vi "03 Channel Tester.vi"(8 "error in (no error)":errorcluster, 11 "Mode":T1(ring)) -> (0 "error out":errorcluster, 2 "CDAQ Data Out":dbl[](array[numeric]))   [LabVIEW 2009]
uses:
  Hybrid Water Heater/Experiments/Sensor.ctl
  <vilib>/DAQmx/read.llb/DAQmx Read (Analog 2D DBL NChan NSamp).vi
  Global Test Variables DPT.vi
  <vilib>/Analysis/NI_AALBase.lvlib
panel:
  in  "CDAQ Data":dbl[](array[numeric])
  in  "Rate":dbl=1000.0
  out "Voltages":dbl[][](graph)
  in  "End":bool
  out "Analog Samples":i32
  in  "I.Bar":i32=5
  out "Bar":cluster{"Mean":dbl, "StdDev":dbl}
  in  "I.Gvol":i32=3
  out "G.Vol":cluster{"Mean":dbl, "StdDev":dbl}
  out "Weight":cluster{"Mean":dbl, "StdDev":dbl}
  in  "I.W":i32=1
  in  "I.Tmp":i32=4
  out "Temp":cluster{"Mean":dbl, "StdDev":dbl}
  out "RH":cluster{"Mean":dbl, "StdDev":dbl}
  in  "I.RH":i32=2
  out "G.Pres.":cluster{"Mean":dbl, "StdDev":dbl}
  in  "I.Gas Pressure":i32
  in  "Timeout":i32=1000
  out "Count":dbl
  out "error gather":errorcluster
  in  "Panel 4":T2[][](array[typedef])=[[{"Mean"=0.0, " Std"=0.0, "Color Box"=8585007}, {"Mean"=0.0, " Std"=0.0, "Color Box"=8585007}, {"Mean"=0.0, " Std"=0.0, "Color Box"=8585007}, {"Mean"=0.0, " Std"=0.0, "Color Box"=8585007}, {"Mean"=0.0, " Std"=0.0, "Color Box"=8585007}, {"Mean"=0.0, " Std"=0.0, "Color Box"=8585007}], [{"Mean"=0.0, " Std"=0.0, "Color Box"=8585007}, {"Mean"=0.0, " Std"=0.0, "Color Box"=8585007}, {"Mean"=0.0, " Std"=0.0, "Color Box"=8585007}, {"Mean"=0.0, " Std"=0.0, "Color Box"=8585007}, {"Mean"=0.0, " Std"=0.0, "Color Box"=8585007}, {"Mean"=0.0, " Std"=0.0, "Color Box"=8585007}], [{"Mean"=0.0, " Std"=0.0, "Color Box"=8585007}, {"Mean"=0.0, " Std"=0.0, "Color Box"=8585007}, {"Mean"=0.0, " Std"=0.0, "Color Box"=8585007}, {"Mean"=0.0, " Std"=0.0, "Color Box"=8585007}, {"Mean"=0.0, " Std"=0.0, "Color Box"=8585007}, {"Mean"=0.0, " Std"=0.0, "Color Box"=8585007}]]
  in  "StDev Thresh":dbl=0.2
  in  "TC Min OK Val":dbl=20.0
  in  "TC Max OK Val":dbl=400.0
  out "Gas Temp":T2={"Mean"=0.0, " Std"=0.0, "Color Box"=8585007}
  in  "Panel 3":T2[][](array[typedef])=[[{"Mean"=0.0, " Std"=0.0, "Color Box"=8585007}, {"Mean"=0.0, " Std"=0.0, "Color Box"=8585007}, {"Mean"=0.0, " Std"=0.0, "Color Box"=8585007}, {"Mean"=0.0, " Std"=0.0, "Color Box"=8585007}, {"Mean"=0.0, " Std"=0.0, "Color Box"=8585007}, {"Mean"=0.0, " Std"=0.0, "Color Box"=8585007}], [{"Mean"=0.0, " Std"=0.0, "Color Box"=8585007}, {"Mean"=0.0, " Std"=0.0, "Color Box"=8585007}, {"Mean"=0.0, " Std"=0.0, "Color Box"=8585007}, {"Mean"=0.0, " Std"=0.0, "Color Box"=8585007}, {"Mean"=0.0, " Std"=0.0, "Color Box"=8585007}, {"Mean"=0.0, " Std"=0.0, "Color Box"=8585007}], [{"Mean"=0.0, " Std"=0.0, "Color Box"=8585007}, {"Mean"=0.0, " Std"=0.0, "Color Box"=8585007}, {"Mean"=0.0, " Std"=0.0, "Color Box"=8585007}, {"Mean"=0.0, " Std"=0.0, "Color Box"=8585007}, {"Mean"=0.0, " Std"=0.0, "Color Box"=8585007}, {"Mean"=0.0, " Std"=0.0, "Color Box"=8585007}]]
  in  "Panel 2":T2[][](array[typedef])=[[{"Mean"=0.0, " Std"=0.0, "Color Box"=8585007}, {"Mean"=0.0, " Std"=0.0, "Color Box"=8585007}, {"Mean"=0.0, " Std"=0.0, "Color Box"=8585007}, {"Mean"=0.0, " Std"=0.0, "Color Box"=8585007}, {"Mean"=0.0, " Std"=0.0, "Color Box"=8585007}, {"Mean"=0.0, " Std"=0.0, "Color Box"=8585007}], [{"Mean"=0.0, " Std"=0.0, "Color Box"=8585007}, {"Mean"=0.0, " Std"=0.0, "Color Box"=8585007}, {"Mean"=0.0, " Std"=0.0, "Color Box"=8585007}, {"Mean"=0.0, " Std"=0.0, "Color Box"=8585007}, {"Mean"=0.0, " Std"=0.0, "Color Box"=8585007}, {"Mean"=0.0, " Std"=0.0, "Color Box"=8585007}], [{"Mean"=0.0, " Std"=0.0, "Color Box"=8585007}, {"Mean"=0.0, " Std"=0.0, "Color Box"=8585007}, {"Mean"=0.0, " Std"=0.0, "Color Box"=8585007}, {"Mean"=0.0, " Std"=0.0, "Color Box"=8585007}, {"Mean"=0.0, " Std"=0.0, "Color Box"=8585007}, {"Mean"=0.0, " Std"=0.0, "Color Box"=8585007}]]
  in  "Panel 1":T2[][](array[typedef])=[[{"Mean"=0.0, " Std"=0.0, "Color Box"=8585007}, {"Mean"=0.0, " Std"=0.0, "Color Box"=8585007}, {"Mean"=0.0, " Std"=0.0, "Color Box"=8585007}, {"Mean"=0.0, " Std"=0.0, "Color Box"=8585007}, {"Mean"=0.0, " Std"=0.0, "Color Box"=8585007}, {"Mean"=0.0, " Std"=0.0, "Color Box"=8585007}], [{"Mean"=0.0, " Std"=0.0, "Color Box"=8585007}, {"Mean"=0.0, " Std"=0.0, "Color Box"=8585007}, {"Mean"=0.0, " Std"=0.0, "Color Box"=8585007}, {"Mean"=0.0, " Std"=0.0, "Color Box"=8585007}, {"Mean"=0.0, " Std"=0.0, "Color Box"=8585007}, {"Mean"=0.0, " Std"=0.0, "Color Box"=8585007}], [{"Mean"=0.0, " Std"=0.0, "Color Box"=8585007}, {"Mean"=0.0, " Std"=0.0, "Color Box"=8585007}, {"Mean"=0.0, " Std"=0.0, "Color Box"=8585007}, {"Mean"=0.0, " Std"=0.0, "Color Box"=8585007}, {"Mean"=0.0, " Std"=0.0, "Color Box"=8585007}, {"Mean"=0.0, " Std"=0.0, "Color Box"=8585007}]]
  in  "Num Samples":i32=5
  in  "Test DAQ":bool
  in  "EXIT":bool
  # "DPT Pannel Channel Tester"
  # "Channel \nGas Pressure 0\nWeight 1\nRH 2\nGas Volume 3\nTemp 4\nBaromentric Pressure 5"
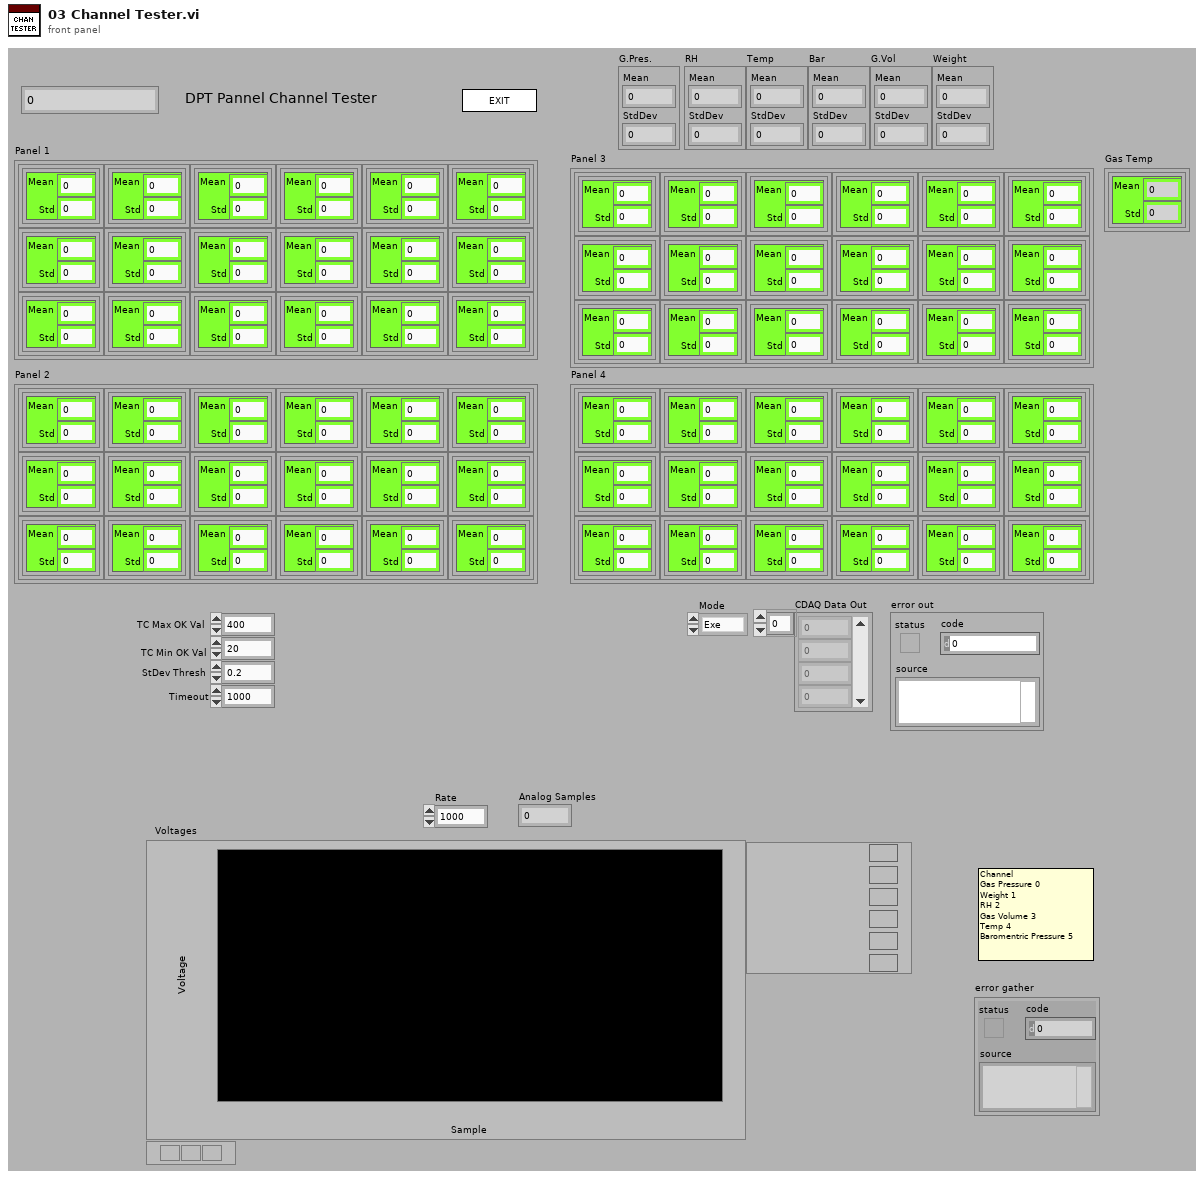
[diagram p1: front panel]
types:
  T1 = enum16{"Exe", "Init CDAQ", "Gather DATA", "Close"}
  T2 = typedef "Sensor.ctl" = cluster{"Mean":dbl, " Std":dbl, "Color Box":u32}
  T3 = enum32{"invalid app kind", "Development System", "Run Time System", "Student Edition", "Embedded LabVIEW", "Evaluation", "Custom"}
  T4 = enum32{"Invalid", "Standard", "Closed", "Hidden", "Minimized", "Maximized"}
  T5 = cluster{"Core":cluster{"Current VI Reference":refnum<vi>, "Close Panel on Exit?":bool}, "Num Samples":i32, "Temp task out":refnum<k21>, "Temp  Data Array":T2[], "AI task out":refnum<k21>, "AI Data":cluster{"Mean":dbl, "StdDev":dbl}[], "Init":bool, "CDAQ Data":dbl[]}
  T6 = cluster{"Current VI Reference":refnum<vi>, "Close Panel on Exit?":bool}
  T7 = typedef "DPT Global Type.ctl" = cluster{"Test Setup":cluster{"3010 resistor":dbl, "Temp Cal":dbl, "Temp Coeff":dbl, "Power On Threshold":dbl, "MA Filter Size":i32, "Weight Offset":dbl, "3011 resistor":dbl, "Gas Enabled":bool, "1020 resistor":dbl, "Scale Com":dbl, "W. Samps":i32}, "Agilent Setup":cluster{"Scale Channel":string, "TC Channels":string, "VDC Discrete Channels":string, "RH Chan":string, "Temp Chan":string, "Tscale Channel":string, "RDB Channel":string, "Gas Temperature":string, "Gas Pressure":string, "Barometric Pressure":string, "Gas Feedback Chan":string}, "Directories":cluster{"Work File Directory":path, "Save File Directory":path, "Library Directory":path, "Data Backup Directory":path}, "Test Information":cluster{"Model:":string, "Temperature:":string, "Engineer:":string, "Technician:":string, "Comments:":string, "Unit:":string, "TR Number:":string, "Test Number:":string, "Test Station:":string, "Empty Dryer Cold Weight:":dbl, "Serial Number:":string, "Build:":string, "Dryer Type":string, "Humidity":string, "Test Title per TR:":string}, "cDAQ Array Locations":cluster{"Scale Channel":string, "TC Channels":string, "VDC Discrete Channel":string, "RH Chan":string, "Temp Chan":string, "Tscale Channel":string, "RDB Channel":string, "Gas Temperature":string, "Gas Pressure":string, "Barometric Pressure":string, "Gas Feedback Chan":string}}
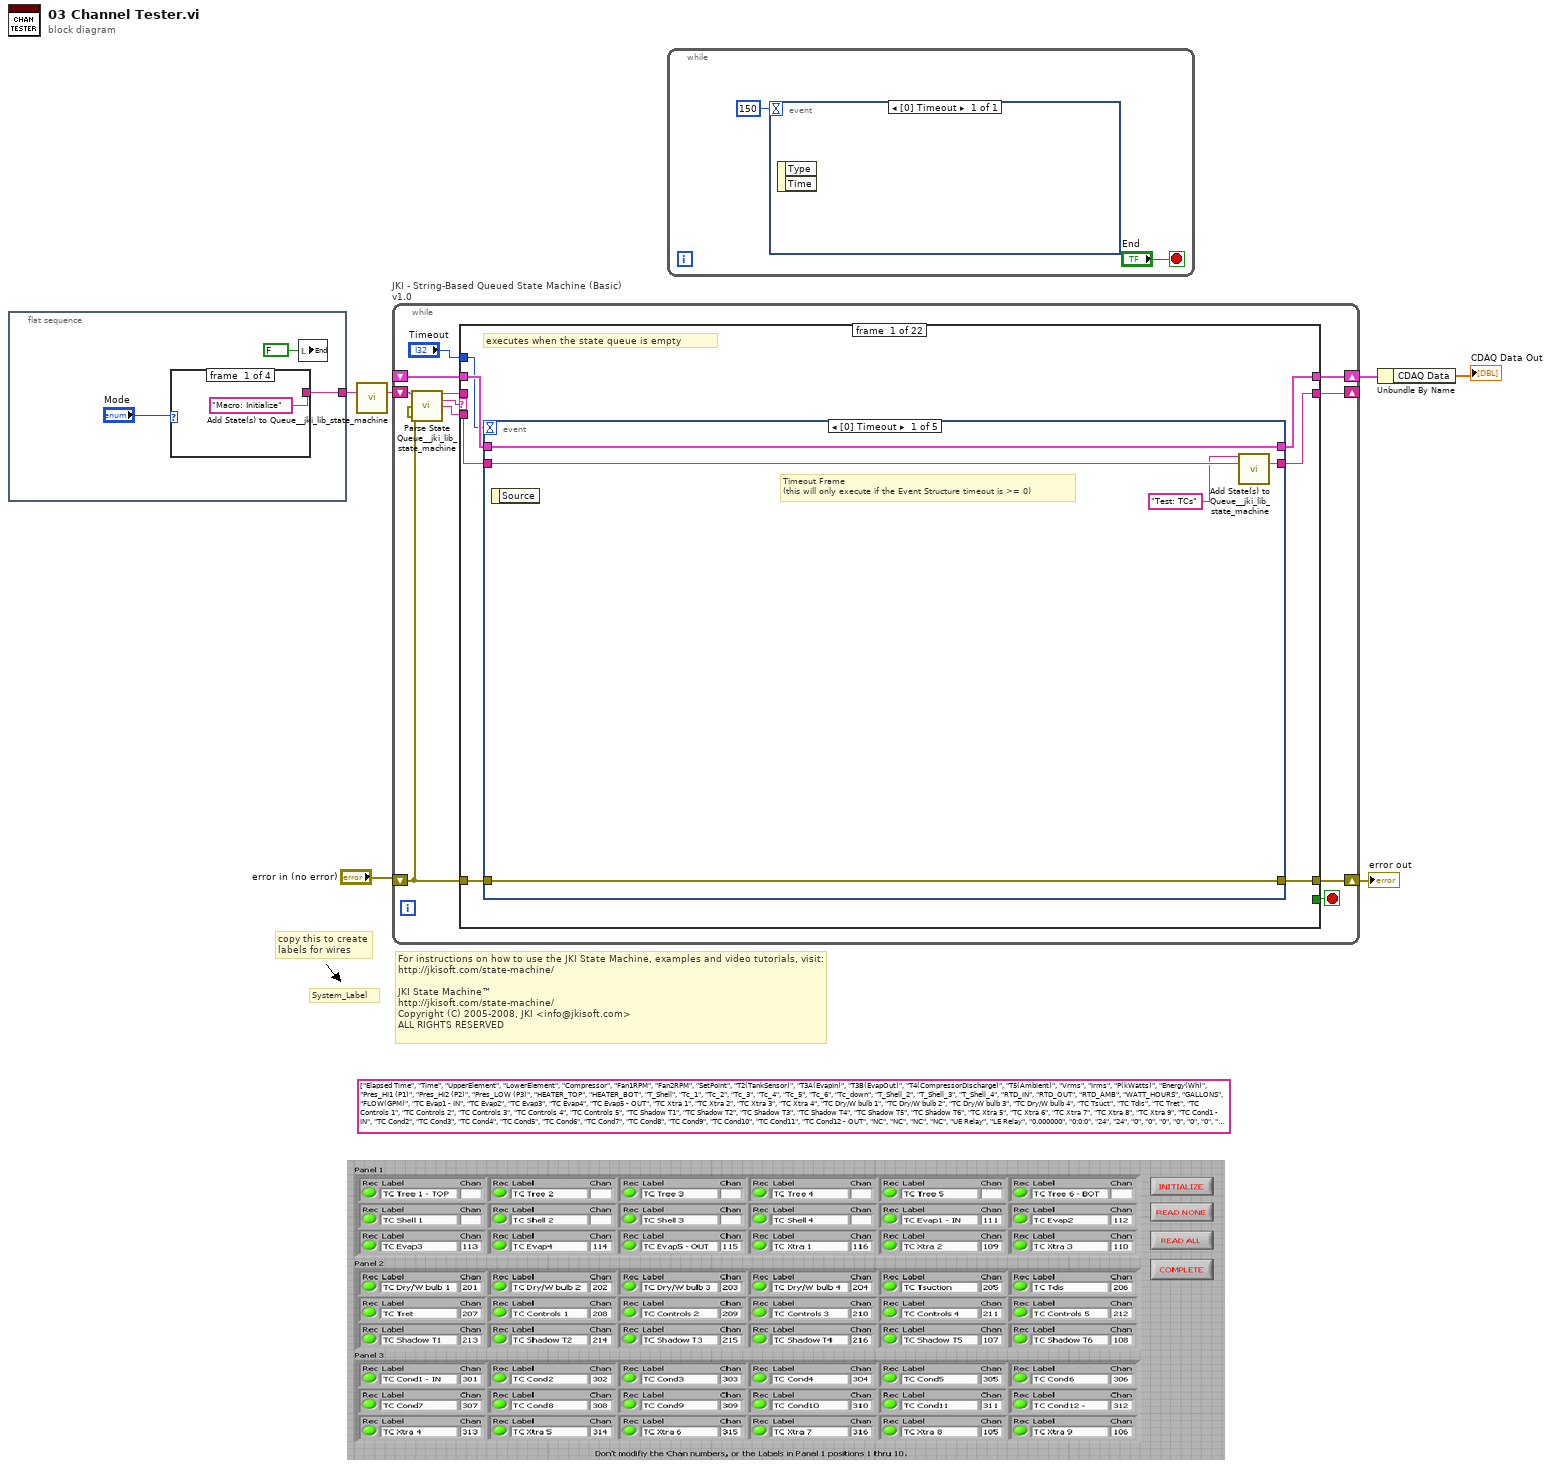
[diagram p0: block diagram]
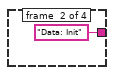
[diagram p2: hidden frame]
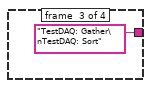
[diagram p3: hidden frame]
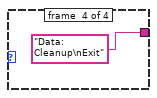
[diagram p4: hidden frame]
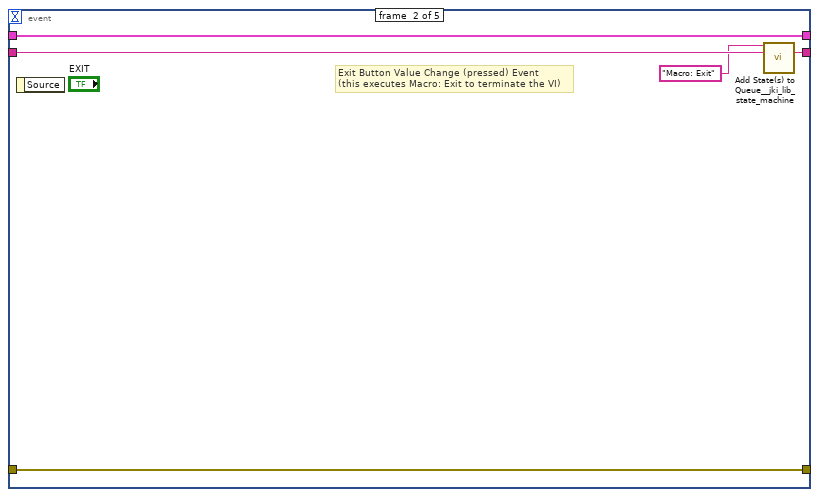
[diagram p5: hidden frame]
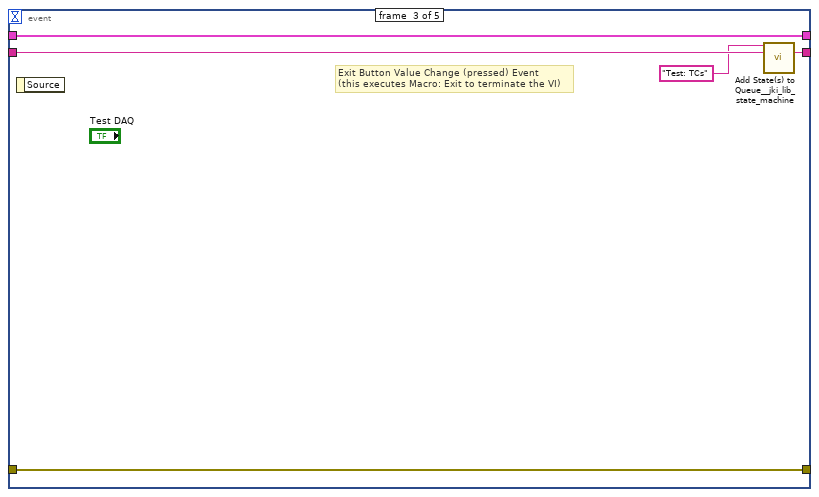
[diagram p6: hidden frame]
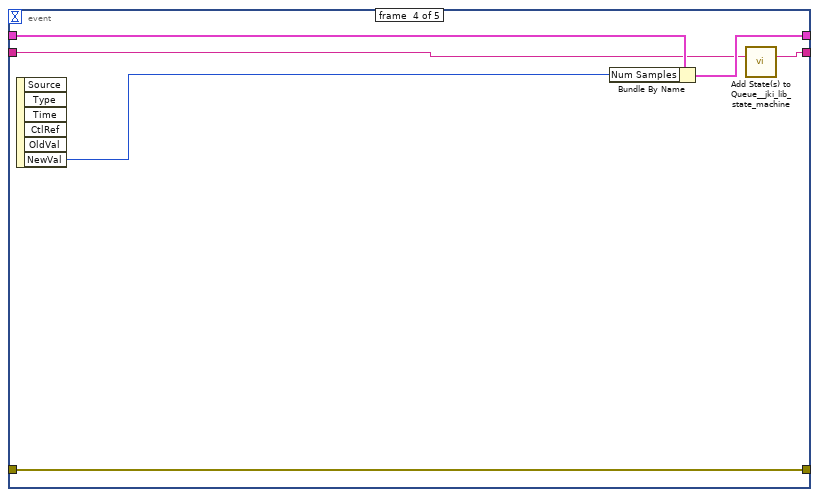
[diagram p7: hidden frame]
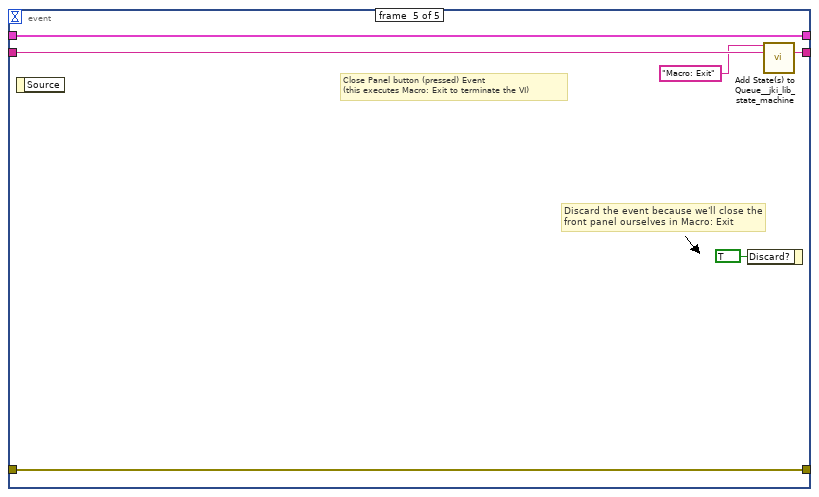
[diagram p8: hidden frame]
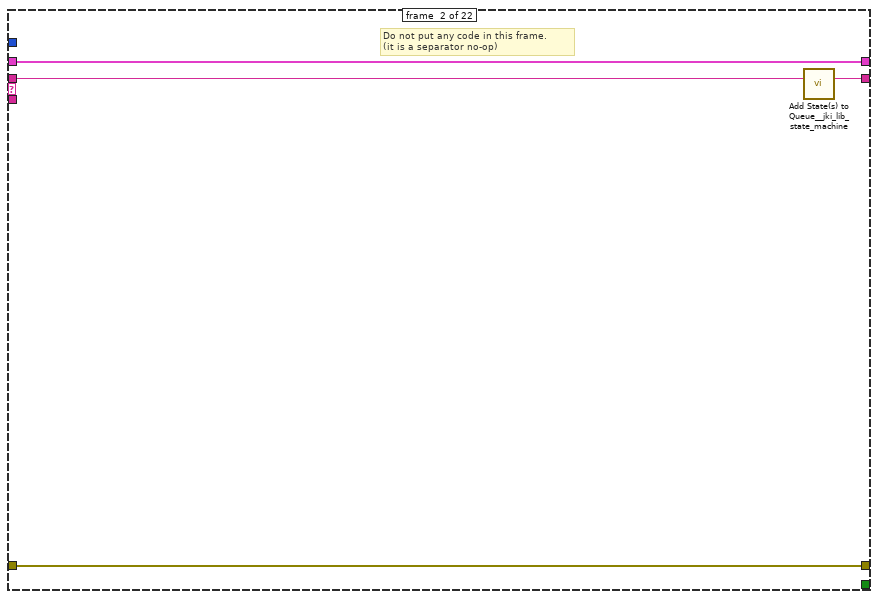
[diagram p9: hidden frame]
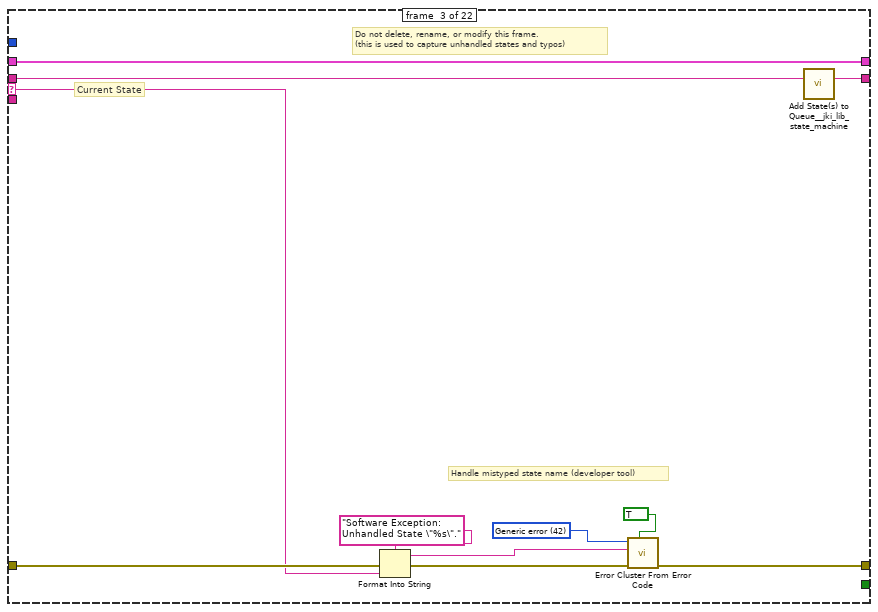
[diagram p10: hidden frame]
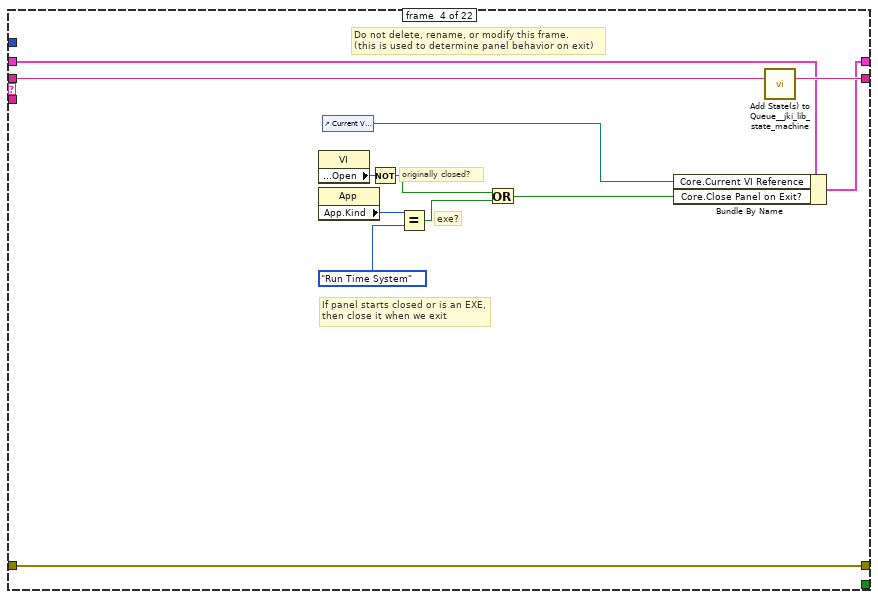
[diagram p11: hidden frame]
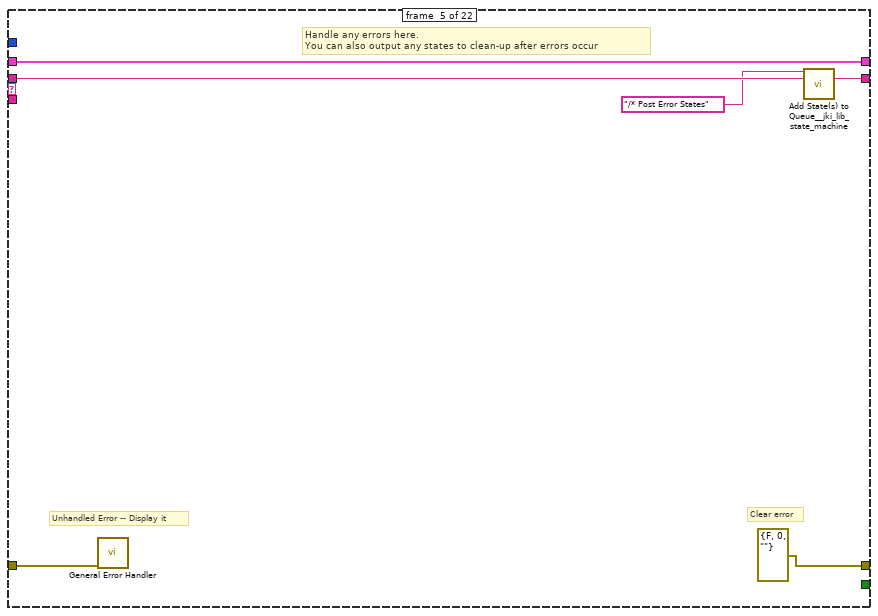
[diagram p12: hidden frame]
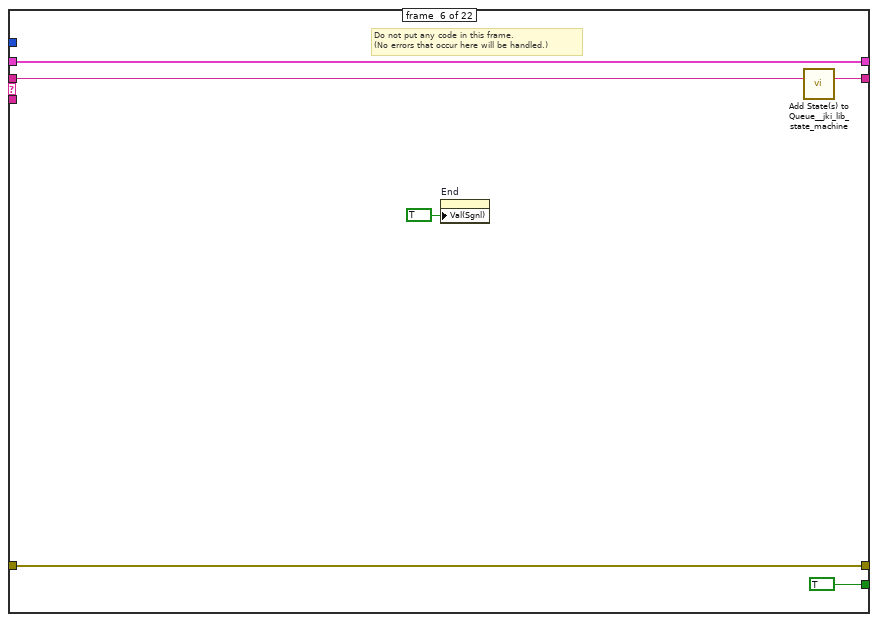
[diagram p13: hidden frame]
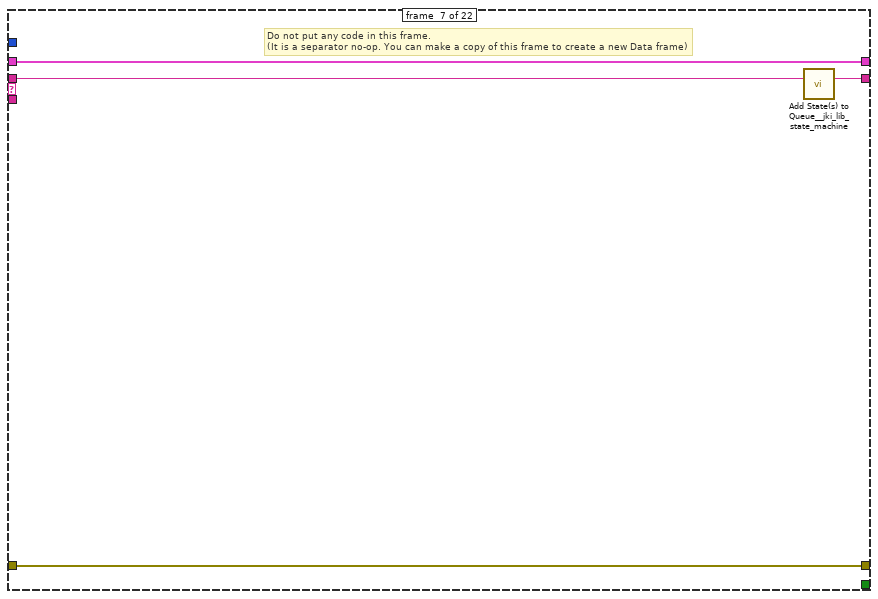
[diagram p14: hidden frame]
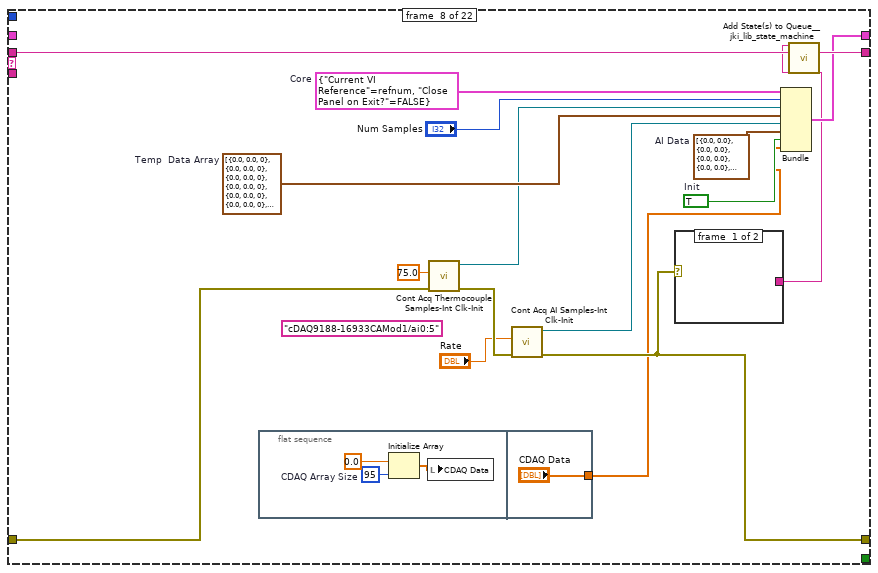
[diagram p15: hidden frame]
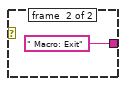
[diagram p16: hidden frame]
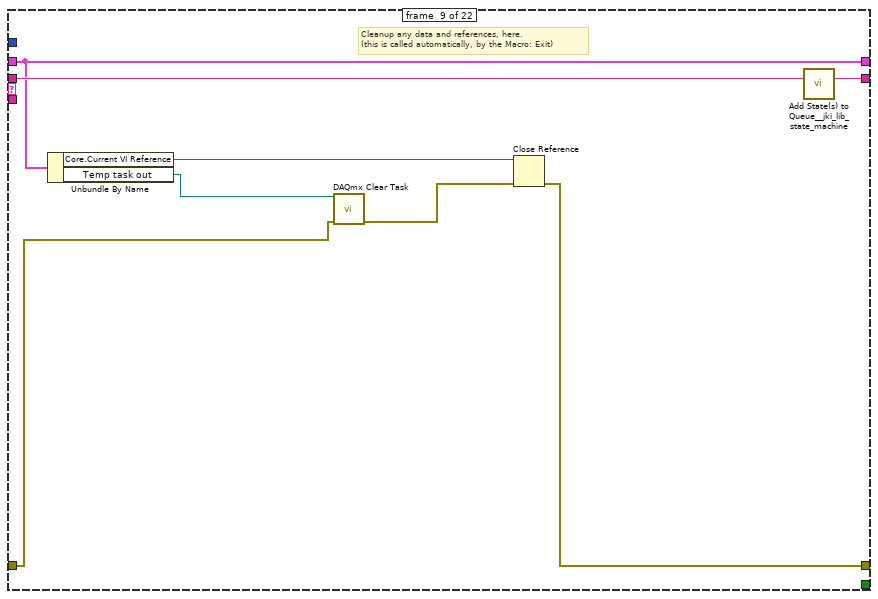
[diagram p17: hidden frame]
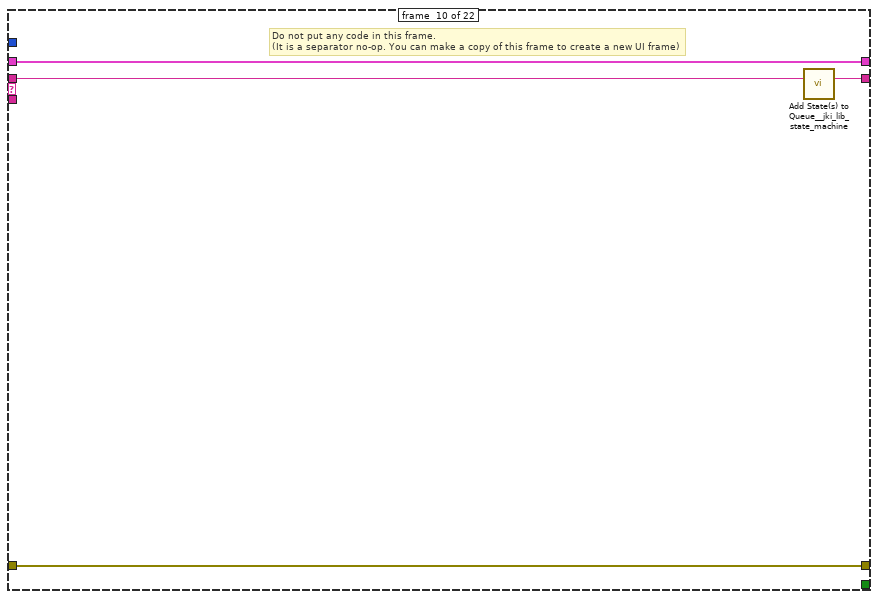
[diagram p18: hidden frame]
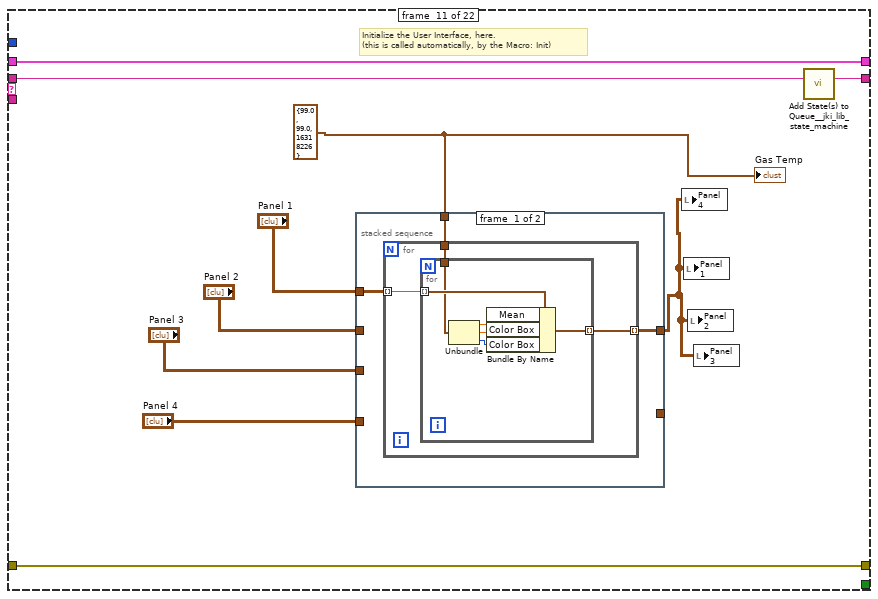
[diagram p19: hidden frame]
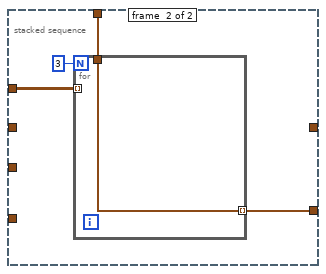
[diagram p20: hidden frame]
diagram:
  (unwired) string[][] [["Elapsed Time", "Time", "UpperElement", "LowerElement", "Compressor", "Fan1RPM", "Fan2RPM", "SetPoint", "T2(TankSensor)", "T3A(EvapIn)", "T3B(EvapOut)", "T4(CompressorDischarge)", "T5(Ambient)", "Vrms", "Irms", "P(kWatts)", "Energy(Wh)", "Pres_HI1 (P1)", "Pres_HI2 (P2)", "Pres_LOW (P3)", "HEATER_TOP", "HEATER_BOT", "T_Shell", "Tc_1", "Tc_2", "Tc_3", "Tc_4", "Tc_5", "Tc_6", "Tc_down", "T_Shell_2", "T_Shell_3", "T_Shell_4", "RTD_IN", "RTD_OUT", "RTD_AMB", "WATT_HOURS", "GALLONS", "FLOW(GPM)", "TC Evap1 - IN", "TC Evap2", "TC Evap3", "TC Evap4", "TC Evap5 - OUT", "TC Xtra 1", "TC Xtra 2", "TC Xtra 3", "TC Xtra 4", "TC Dry/W bulb 1", "TC Dry/W bulb 2", "TC Dry/W bulb 3", "TC Dry/W bulb 4", "TC Tsuct", "TC Tdis", "TC Tret", "TC Controls 1", "TC Controls 2", "TC Controls 3", "TC Controls 4", "TC Controls 5", "TC Shadow T1", "TC Shadow T2", "TC Shadow T3", "TC Shadow T4", "TC Shadow T5", "TC Shadow T6", "TC Xtra 5", "TC Xtra 6", "TC Xtra 7", "TC Xtra 8", "TC Xtra 9", "TC Cond1 - IN", "TC Cond2", "TC Cond3", "TC Cond4", "TC Cond5", "TC Cond6", "TC Cond7", "TC Cond8", "TC Cond9", "TC Cond10", "TC Cond11", "TC Cond12 - OUT", "NC", "NC", "NC", "NC", "UE Relay", "LE Relay"], ["0.000000", "0:0:0", "24", "24", "0", "0", "0", "0", "0", "0", "0", "0", "0", "-229.980000", "-0.000013", "0.003000", "0.000000", "68.20", "67.08", "68.20", "1.00", "1.00", "214745087.90", "63.60", "63.80", "63.90", "63.70", "63.60", "63.90", "69.60", "-322.40", "-318.30", "-214738534.30", "-214738534.30", "-214738534.30", "52.30", "0.00", "0.30", "0.00", "534.04", "-178199999999999999000000000000000000000.00", "55.58", "55.35", "57.06", "55.53", "55.22", "-178199999999999999000000000000000000000.00", "-178199999999999999000000000000000000000.00", "53.73", "54.09", "-178199999999999999000000000000000000000.00", "-178199999999999999000000000000000000000.00", "303.05", "-178199999999999999000000000000000000000.00", "178199999999999999000000000000000000000.00", "-178199999999999999000000000000000000000.00", "460.73", "626.99", "-178199999999999999000000000000000000000.00", "178199999999999999000000000000000000000.00", "-178199999999999999000000000000000000000.00", "131.37", "178199999999999999000000000000000000000.00", "-178199999999999999000000000000000000000.00", "-178199999999999999000000000000000000000.00", "409.13", "259.86", "-178199999999999999000000000000000000000.00", "178199999999999999000000000000000000000.00", "-178199999999999999000000000000000000000.00", "-57.06", "62.09", "61.89", "61.87", "62.14", "62.63", "178199999999999999000000000000000000000.00", "-178199999999999999000000000000000000000.00", "178199999999999999000000000000000000000.00", "-70.58", "-178199999999999999000000000000000000000.00", "178199999999999999000000000000000000000.00", "-178199999999999999000000000000000000000.00", "393.52", "116.86", "83.34", "59.96", "0", "0"]] ("Output Data")
  # "For instructions on how to use the JKI State Machine, examples and video tutorials, visit:\nhttp://jkisoft.com/state-machine/\n\nJKI State Machine™\nhttp://jkisoft.com/state-machine/\nCopyright (C) 2005-2008, JKI <info@jkisoft.com>\nALL RIGHTS RESERVED"
  # "copy this to create labels for wires"
  # "System_Label"
  n1 = flat-sequence {
    tunnel: [w9] -> w5
    frame #0 {
      n2 = case shown="\"Close\"" "Mode" {
        tunnel: ["Macro: Initialize" "Data: Init" "TestDAQ: Gather\nTestDAQ: Sort" "Data: Cleanup\nExit"] -> w9
        frame #0 {
        }
        frame #1 {
        }
        frame #2 {
        }
        frame #3 {
        }
      }
      n3 = local write "End"(FALSE ("stop")) -> ()
    }
  }
  n4 = call <vilib>:"Add State(s) to Queue__jki_lib_state_machine.vi"("State(s) in (\"\")"=w5) -> ("States Out"=w6:string)  [unwired: 14 in]
  n5 = while "JKI - String-Based Queued State Machine (Basic) v1.0" {
    shift-right: [w17] -> w2
    shift-left: _ -> [w16]
    shift-right: [w20] -> w3
    shift-left: "error in (no error)" -> [w14]
    shift-right: [w19] -> _
    shift-left: w6 -> [w21]
    stop <- w18 stop-if-true
    n6 = call <vilib>:"Parse State Queue__jki_lib_state_machine.vi"("State Queue"=w21, "Error In (no error)"=w14) -> ("Remaining States"=w23:string, "Current State"=w24:string, "Arguments"=w22:string)  [unwired: 11 in]
    n7 = case shown="\"Data: Initialize\"" w24 {
      selector: w24 -> [_ _ w63 _ _ _ _ _ _ _ _ _ _ _ _ _ _ _ _ _ _ _]
      tunnel: w23 -> [w31 w62 w67 w85 w91 w97 w101 w118 w131 w135 w145 w168 w179 w205 w210 w220 w224 w229 w233 w252 w279 w487]
      tunnel: w22 -> [_ _ _ _ _ _ _ _ _ _ _ w163 w173 _ _ _ _ _ _ _ _ _]
      tunnel: w16 -> [w29 w59 w65 w76 w88 w95 w98 _ w127 w132 w143 w166 w175 w202 w207 w217 w221 w227 w230 w250 w273 w484]
      tunnel: [w28 w60 w69 w82 errorcluster {"status"=FALSE, "code"=0, "source"=""} ("error out") w94 w99 w105 w128 w133 w142 w164 w176 w203 w208 w218 w222 w225 w231 w244 w277 w485] -> w20
      tunnel: w14 -> [w27 w60 w68 w82 w87 w94 w99 w110 w125 w133 w142 w165 w177 w203 w208 w218 w222 w225 w231 w247 w277 w485]
      tunnel: [w30 w61 w66 w84 w90 w96 w100 w117 w130 w134 w144 w167 w178 w204 w209 w219 w223 w228 w232 w251 w278 w486] -> w19
      tunnel: [_ _ _ _ _ TRUE _ _ _ _ _ _ _ _ _ _ _ _ _ _ _ _] -> w18
      tunnel: [w26 w59 w65 w83 w88 w95 w98 w116 w127 w132 w143 w166 w175 w202 w207 w217 w221 w227 w230 w248 w272 w484] -> w17
      tunnel: "Timeout" -> [w25 _ _ _ _ _ _ _ _ _ _ _ _ _ _ _ _ _ _ _ _ _]
      frame #0 {
        # "executes when the state queue is empty"
        n8 = event shown="[0] Timeout" {
          selector: _ -> [_ _ _ _ _]
          dyn-events: _ -> [_ _ _ _ _]
          timeout: w25 -> [_ _ _ _ _]
          tunnel: w31 -> [w36 w41 w46 w50 w58]
          tunnel: [w35 w40 w45 w49 w57] -> w30
          tunnel: w29 -> [w33 w38 w43 w52 w55]
          tunnel: [w34 w39 w44 w48 w56] -> w28
          tunnel: w27 -> [w34 w39 w44 w48 w56]
          tunnel: [w33 w38 w43 w51 w55] -> w26
          event #0 {
            # "Timeout Frame\n(this will only execute if the Event Structure timeout is >= 0)"
            n9 = event-data() -> ()  [unwired: 1 in, 1 out]
            n10 = call <vilib>:"Add State(s) to Queue__jki_lib_state_machine.vi"("State(s) in Front (\"\")"="Test: TCs", "State(s) in (\"\")"=w36) -> ("States Out"=w35:string)  [unwired: 13 in]
          }
          event #1 {
            # "Exit Button Value Change (pressed) Event\n(this executes Macro: Exit to terminate the VI)"
            n11 = event-data() -> ()  [unwired: 1 in, 1 out]
            n12 = call <vilib>:"Add State(s) to Queue__jki_lib_state_machine.vi"("State(s) in Front (\"\")"="Macro: Exit", "State(s) in (\"\")"=w41) -> ("States Out"=w40:string)  [unwired: 13 in]
          }
          event #2 {
            # "Exit Button Value Change (pressed) Event\n(this executes Macro: Exit to terminate the VI)"
            n13 = event-data() -> ()  [unwired: 1 in, 1 out]
            n14 = call <vilib>:"Add State(s) to Queue__jki_lib_state_machine.vi"("State(s) in Front (\"\")"="Test: TCs", "State(s) in (\"\")"=w46) -> ("States Out"=w45:string)  [unwired: 13 in]
          }
          event #3 {
            n15 = event-data() -> ("NewVal"=w47:i32)  [unwired: 1 in, 5 out]
            n16 = Bundle By Name(cluster=w52, "Num Samples"=w47) -> (w51:T5)
            n17 = call <vilib>:"Add State(s) to Queue__jki_lib_state_machine.vi"("State(s) in (\"\")"=w50) -> ("States Out"=w49:string)  [unwired: 14 in]
          }
          event #4 {
            # "Discard the event because we'll close the front panel ourselves in Macro: Exit"
            # "Close Panel button (pressed) Event\n(this executes Macro: Exit to terminate the VI)"
            n18 = event-data() -> ()  [unwired: 1 in, 1 out]
            n19 = event-data("Discard?"=TRUE) -> ()  [unwired: 1 in, 1 out]
            n20 = call <vilib>:"Add State(s) to Queue__jki_lib_state_machine.vi"("State(s) in Front (\"\")"="Macro: Exit", "State(s) in (\"\")"=w58) -> ("States Out"=w57:string)  [unwired: 13 in]
          }
        }
      }
      frame #1 {
        # "Do not put any code in this frame.\n(it is a separator no-op)"
        n21 = call <vilib>:"Add State(s) to Queue__jki_lib_state_machine.vi"("State(s) in (\"\")"=w62) -> ("States Out"=w61:string)  [unwired: 14 in]
      }
      frame #2 {
        w72 = 42 items=["No error", "Argument error", "Memory is full", "Out of zone", "End of file", "File already open", "Generic file I/O error", "File not found", "File permission error", "Disk is full", "Duplicate path", "Too many files open", "System feature not enabled", "Resource file not found", "Cannot add resource", "Resource not found", "Image not found", "Image memory error", "Pen does not exist", "Config type invalid", "Config token not found", "Config parse error", "Config memory error", "Bad external code format", "Bad external code offset", "External code not present", "Null window", "Destroy window error", "Null menu", "Print aborted", "Bad print record", "Print driver error", "Windows error during printing", "Memory error during printing", "Print dialog error", "Generic print error", "Invalid device refnum", "Device not found", "Device parameter error", "Device unit error", "Cannot open device", "Device call aborted", "Generic error", "Cancelled by user", "Object ID too low", "Object ID too high", "Object not in heap", "Unknown heap", "Unknown object (invalid DefProc)", "Unknown object (DefProc not in table)", "Message out of range", "Invalid (null) method", "Unknown message", "Manager call not supported", "Bad address", "Network operation in progress", "Network operation timed out", "Connection is busy", "Network attribute not supported", "Network error", "Address in use", "System out of memory", "Connection aborted", "Connection refused", "Not connected", "Already connected", "Connection closed", "Initialization error (interapplication manager)", "Bad occurrence", "Wait on unbound occurrence handler", "Occurrence queue overflow", "Datalog type conflict", "Unused", "Unrecognized type (interapplication manager)", "Memory corrupt", "Failed to make temporary DLL", "Old CIN version", "Drag socket not found", "Failed to load drop-object", "Failed to register OLE object", "Failed to release OLE object", "Format specifier type mismatch", "Unknown format specifier", "Too few format specifiers", "Too many format specifiers", "Scan failed", "Newer CIN version", "Error converting to variant", "Runtime menu error", "Password tampered", "Variant attribute not found", "Incompatible variant data type", "Event data is not available", "Event Store is not present", "Occurrence is not found", "Event Queue is not created", "Event info is not available", "Refnum passed is NULL", "Error retrieving Class GUID", "Error retrieving CoClass GUID", "Error retrieving TypeLib GUID.", "Bad built application magic bytes.", "Specific driver is different from the specific driver associated with the Logical Name.", "There is no session opened to the class driver.", "Max Error", "MAX - Error with config objects", "MAX - Error loading configuration", "MAX - Group not supported"]
        # "Current State"
        # "Do not delete, rename, or modify this frame.\n(this is used to capture unhandled states and typos)"
        # "Handle mistyped state name (developer tool)"
        n22 = Format Into String(format string="Software Exception: Unhandled State \"%s\"." ("message"), error in=w68, w63) -> (resulting string=w71:string, error out=w70:errorcluster)  [unwired: 1 in]
        n23 = call <vilib>:"Error Cluster From Error Code.vi"("show call chain? (False)"=TRUE, "error in (no error)"=w70, "error message (\"\")"=w71, "error code (0)"=w72) -> ("error out"=w69:errorcluster)  [unwired: 5 in]
        n24 = call <vilib>:"Add State(s) to Queue__jki_lib_state_machine.vi"("State(s) in (\"\")"=w67) -> ("States Out"=w66:string)  [unwired: 14 in]
      }
      frame #3 {
        # "Do not delete, rename, or modify this frame.\n(this is used to determine panel behavior on exit)"
        # "originally closed?"
        # "exe?"
        # "If panel starts closed or is an EXE, then close it when we exit"
        n25 = property class="VI"() -> ("Front Panel.Open"=w81:bool)  [unwired: 2 in, 2 out]
        n26 = property class="App"() -> ("App.Kind"=w80:T3)  [unwired: 2 in, 2 out]
        n27 = control-ref of="Current VI Reference"() -> (w74:refnum<vi>)
        n28 = Not(x=w81) -> (.not. x?=w78:bool)
        n29 = Equal?(x=w80, y=T3."Run Time System" ("Application:Kind")) -> (x = y?=w77:bool)
        n30 = Or(x=w78, y=w77) -> (x .or. y?=w75:bool)
        n31 = Bundle By Name(cluster=w76, "Core.Current VI Reference"=w74, "Core.Close Panel on Exit?"=w75) -> (w83:T5)
        n32 = call <vilib>:"Add State(s) to Queue__jki_lib_state_machine.vi"("State(s) in (\"\")"=w85) -> ("States Out"=w84:string)  [unwired: 14 in]
      }
      frame #4 {
        # "Unhandled Error -- Display it"
        # "Handle any errors here.\nYou can also output any states to clean-up after errors occur"
        # "Clear error"
        n33 = call <vilib>:"General Error Handler.vi"("error in (no error)"=w87) -> ()  [unwired: 10 in, 5 out]
        n34 = call <vilib>:"Add State(s) to Queue__jki_lib_state_machine.vi"("State(s) in Front (\"\")"="/* Post Error States", "State(s) in (\"\")"=w91) -> ("States Out"=w90:string)  [unwired: 13 in]
      }
      frame #5 {
        # "Do not put any code in this frame.\n(No errors that occur here will be handled.)"
        n35 = property on="End" class="Bool (strict)"("Val(Sgnl)"=TRUE ("Value (Signaling)")) -> ()  [unwired: 2 in, 2 out]
        n36 = call <vilib>:"Add State(s) to Queue__jki_lib_state_machine.vi"("State(s) in (\"\")"=w97) -> ("States Out"=w96:string)  [unwired: 14 in]
      }
      frame #6 {
        # "Do not put any code in this frame.\n(It is a separator no-op. You can make a copy of this frame to create a new Data frame)"
        n37 = call <vilib>:"Add State(s) to Queue__jki_lib_state_machine.vi"("State(s) in (\"\")"=w101) -> ("States Out"=w100:string)  [unwired: 14 in]
      }
      frame #7 {
        w103 = TRUE  # Init
        (unwired) "cDAQ9188-16933CAMod1/ai0:5"
        w107 = cluster{"Mean":dbl, "StdDev":dbl}[] [{"Mean"=0.0, "StdDev"=0.0}, {"Mean"=0.0, "StdDev"=0.0}, {"Mean"=0.0, "StdDev"=0.0}, {"Mean"=0.0, "StdDev"=0.0}, {"Mean"=0.0, "StdDev"=0.0}, {"Mean"=0.0, "StdDev"=0.0}, {"Mean"=0.0, "StdDev"=0.0}, {"Mean"=0.0, "StdDev"=0.0}, {"Mean"=0.0, "StdDev"=0.0}, {"Mean"=0.0, "StdDev"=0.0}, {"Mean"=0.0, "StdDev"=0.0}, {"Mean"=0.0, "StdDev"=0.0}, {"Mean"=0.0, "StdDev"=0.0}, {"Mean"=0.0, "StdDev"=0.0}, {"Mean"=0.0, "StdDev"=0.0}, {"Mean"=0.0, "StdDev"=0.0}]  # AI Data
        w113 = T2[] [{"Mean"=0.0, " Std"=0.0, "Color Box"=0}, {"Mean"=0.0, " Std"=0.0, "Color Box"=0}, {"Mean"=0.0, " Std"=0.0, "Color Box"=0}, {"Mean"=0.0, " Std"=0.0, "Color Box"=0}, {"Mean"=0.0, " Std"=0.0, "Color Box"=0}, {"Mean"=0.0, " Std"=0.0, "Color Box"=0}, {"Mean"=0.0, " Std"=0.0, "Color Box"=0}, {"Mean"=0.0, " Std"=0.0, "Color Box"=0}, {"Mean"=0.0, " Std"=0.0, "Color Box"=0}, {"Mean"=0.0, " Std"=0.0, "Color Box"=0}, {"Mean"=0.0, " Std"=0.0, "Color Box"=0}, {"Mean"=0.0, " Std"=0.0, "Color Box"=0}, {"Mean"=0.0, " Std"=0.0, "Color Box"=0}, {"Mean"=0.0, " Std"=0.0, "Color Box"=0}, {"Mean"=0.0, " Std"=0.0, "Color Box"=0}, {"Mean"=0.0, " Std"=0.0, "Color Box"=0}, {"Mean"=0.0, " Std"=0.0, "Color Box"=0}, {"Mean"=0.0, " Std"=0.0, "Color Box"=0}, {"Mean"=0.0, " Std"=0.0, "Color Box"=0}, {"Mean"=0.0, " Std"=0.0, "Color Box"=0}, {"Mean"=0.0, " Std"=0.0, "Color Box"=0}, {"Mean"=0.0, " Std"=0.0, "Color Box"=0}, {"Mean"=0.0, " Std"=0.0, "Color Box"=0}, {"Mean"=0.0, " Std"=0.0, "Color Box"=0}, {"Mean"=0.0, " Std"=0.0, "Color Box"=0}, {"Mean"=0.0, " Std"=0.0, "Color Box"=0}, {"Mean"=0.0, " Std"=0.0, "Color Box"=0}, {"Mean"=0.0, " Std"=0.0, "Color Box"=0}, {"Mean"=0.0, " Std"=0.0, "Color Box"=0}, {"Mean"=0.0, " Std"=0.0, "Color Box"=0}, {"Mean"=0.0, " Std"=0.0, "Color Box"=0}, {"Mean"=0.0, " Std"=0.0, "Color Box"=0}, {"Mean"=0.0, " Std"=0.0, "Color Box"=0}, {"Mean"=0.0, " Std"=0.0, "Color Box"=0}, {"Mean"=0.0, " Std"=0.0, "Color Box"=0}, {"Mean"=0.0, " Std"=0.0, "Color Box"=0}, {"Mean"=0.0, " Std"=0.0, "Color Box"=0}, {"Mean"=0.0, " Std"=0.0, "Color Box"=0}, {"Mean"=0.0, " Std"=0.0, "Color Box"=0}, {"Mean"=0.0, " Std"=0.0, "Color Box"=0}, {"Mean"=0.0, " Std"=0.0, "Color Box"=0}, {"Mean"=0.0, " Std"=0.0, "Color Box"=0}, {"Mean"=0.0, " Std"=0.0, "Color Box"=0}, {"Mean"=0.0, " Std"=0.0, "Color Box"=0}, {"Mean"=0.0, " Std"=0.0, "Color Box"=0}, {"Mean"=0.0, " Std"=0.0, "Color Box"=0}, {"Mean"=0.0, " Std"=0.0, "Color Box"=0}, {"Mean"=0.0, " Std"=0.0, "Color Box"=0}, {"Mean"=0.0, " Std"=0.0, "Color Box"=0}, {"Mean"=0.0, " Std"=0.0, "Color Box"=0}, {"Mean"=0.0, " Std"=0.0, "Color Box"=0}, {"Mean"=0.0, " Std"=0.0, "Color Box"=0}, {"Mean"=0.0, " Std"=0.0, "Color Box"=0}, {"Mean"=0.0, " Std"=0.0, "Color Box"=0}, {"Mean"=0.0, " Std"=0.0, "Color Box"=0}, {"Mean"=0.0, " Std"=0.0, "Color Box"=0}, {"Mean"=0.0, " Std"=0.0, "Color Box"=0}, {"Mean"=0.0, " Std"=0.0, "Color Box"=0}, {"Mean"=0.0, " Std"=0.0, "Color Box"=0}, {"Mean"=0.0, " Std"=0.0, "Color Box"=0}, {"Mean"=0.0, " Std"=0.0, "Color Box"=0}, {"Mean"=0.0, " Std"=0.0, "Color Box"=0}, {"Mean"=0.0, " Std"=0.0, "Color Box"=0}, {"Mean"=0.0, " Std"=0.0, "Color Box"=0}, {"Mean"=0.0, " Std"=0.0, "Color Box"=0}, {"Mean"=0.0, " Std"=0.0, "Color Box"=0}, {"Mean"=0.0, " Std"=0.0, "Color Box"=0}, {"Mean"=0.0, " Std"=0.0, "Color Box"=0}, {"Mean"=0.0, " Std"=0.0, "Color Box"=0}, {"Mean"=0.0, " Std"=0.0, "Color Box"=0}, {"Mean"=0.0, " Std"=0.0, "Color Box"=0}, {"Mean"=0.0, " Std"=0.0, "Color Box"=0}, {"Mean"=0.0, " Std"=0.0, "Color Box"=0}, {"Mean"=0.0, " Std"=0.0, "Color Box"=0}, {"Mean"=0.0, " Std"=0.0, "Color Box"=0}, {"Mean"=0.0, " Std"=0.0, "Color Box"=0}, {"Mean"=0.0, " Std"=0.0, "Color Box"=0}, {"Mean"=0.0, " Std"=0.0, "Color Box"=0}, {"Mean"=0.0, " Std"=0.0, "Color Box"=0}, {"Mean"=0.0, " Std"=0.0, "Color Box"=0}, {"Mean"=0.0, " Std"=0.0, "Color Box"=0}, {"Mean"=0.0, " Std"=0.0, "Color Box"=0}, {"Mean"=0.0, " Std"=0.0, "Color Box"=0}, {"Mean"=0.0, " Std"=0.0, "Color Box"=0}, {"Mean"=0.0, " Std"=0.0, "Color Box"=0}, {"Mean"=0.0, " Std"=0.0, "Color Box"=0}, {"Mean"=0.0, " Std"=0.0, "Color Box"=0}, {"Mean"=0.0, " Std"=0.0, "Color Box"=0}, {"Mean"=0.0, " Std"=0.0, "Color Box"=0}, {"Mean"=0.0, " Std"=0.0, "Color Box"=0}, {"Mean"=0.0, " Std"=0.0, "Color Box"=0}, {"Mean"=0.0, " Std"=0.0, "Color Box"=0}, {"Mean"=0.0, " Std"=0.0, "Color Box"=0}, {"Mean"=0.0, " Std"=0.0, "Color Box"=0}, {"Mean"=0.0, " Std"=0.0, "Color Box"=0}, {"Mean"=0.0, " Std"=0.0, "Color Box"=0}, {"Mean"=0.0, " Std"=0.0, "Color Box"=0}, {"Mean"=0.0, " Std"=0.0, "Color Box"=0}, {"Mean"=0.0, " Std"=0.0, "Color Box"=0}, {"Mean"=0.0, " Std"=0.0, "Color Box"=0}, {"Mean"=0.0, " Std"=0.0, "Color Box"=0}, {"Mean"=0.0, " Std"=0.0, "Color Box"=0}, {"Mean"=0.0, " Std"=0.0, "Color Box"=0}, {"Mean"=0.0, " Std"=0.0, "Color Box"=0}, {"Mean"=0.0, " Std"=0.0, "Color Box"=0}, {"Mean"=0.0, " Std"=0.0, "Color Box"=0}, {"Mean"=0.0, " Std"=0.0, "Color Box"=0}, {"Mean"=0.0, " Std"=0.0, "Color Box"=0}, {"Mean"=0.0, " Std"=0.0, "Color Box"=0}, {"Mean"=0.0, " Std"=0.0, "Color Box"=0}, {"Mean"=0.0, " Std"=0.0, "Color Box"=0}, {"Mean"=0.0, " Std"=0.0, "Color Box"=0}, {"Mean"=0.0, " Std"=0.0, "Color Box"=0}, {"Mean"=0.0, " Std"=0.0, "Color Box"=0}, {"Mean"=0.0, " Std"=0.0, "Color Box"=0}, {"Mean"=0.0, " Std"=0.0, "Color Box"=0}, {"Mean"=0.0, " Std"=0.0, "Color Box"=0}, {"Mean"=0.0, " Std"=0.0, "Color Box"=0}, {"Mean"=0.0, " Std"=0.0, "Color Box"=0}, {"Mean"=0.0, " Std"=0.0, "Color Box"=0}, {"Mean"=0.0, " Std"=0.0, "Color Box"=0}, {"Mean"=0.0, " Std"=0.0, "Color Box"=0}, {"Mean"=0.0, " Std"=0.0, "Color Box"=0}, {"Mean"=0.0, " Std"=0.0, "Color Box"=0}, {"Mean"=0.0, " Std"=0.0, "Color Box"=0}, {"Mean"=0.0, " Std"=0.0, "Color Box"=0}, {"Mean"=0.0, " Std"=0.0, "Color Box"=0}, {"Mean"=0.0, " Std"=0.0, "Color Box"=0}, {"Mean"=0.0, " Std"=0.0, "Color Box"=0}, {"Mean"=0.0, " Std"=0.0, "Color Box"=0}, {"Mean"=0.0, " Std"=0.0, "Color Box"=0}, {"Mean"=0.0, " Std"=0.0, "Color Box"=0}, {"Mean"=0.0, " Std"=0.0, "Color Box"=0}, {"Mean"=0.0, " Std"=0.0, "Color Box"=0}, {"Mean"=0.0, " Std"=0.0, "Color Box"=0}, {"Mean"=0.0, " Std"=0.0, "Color Box"=0}, {"Mean"=0.0, " Std"=0.0, "Color Box"=0}, {"Mean"=0.0, " Std"=0.0, "Color Box"=0}, {"Mean"=0.0, " Std"=0.0, "Color Box"=0}, {"Mean"=0.0, " Std"=0.0, "Color Box"=0}, {"Mean"=0.0, " Std"=0.0, "Color Box"=0}, {"Mean"=0.0, " Std"=0.0, "Color Box"=0}, {"Mean"=0.0, " Std"=0.0, "Color Box"=0}, {"Mean"=0.0, " Std"=0.0, "Color Box"=0}, {"Mean"=0.0, " Std"=0.0, "Color Box"=0}, {"Mean"=0.0, " Std"=0.0, "Color Box"=0}, {"Mean"=0.0, " Std"=0.0, "Color Box"=0}, {"Mean"=0.0, " Std"=0.0, "Color Box"=0}, {"Mean"=0.0, " Std"=0.0, "Color Box"=0}, {"Mean"=0.0, " Std"=0.0, "Color Box"=0}, {"Mean"=0.0, " Std"=0.0, "Color Box"=0}, {"Mean"=0.0, " Std"=0.0, "Color Box"=0}, {"Mean"=0.0, " Std"=0.0, "Color Box"=0}, {"Mean"=0.0, " Std"=0.0, "Color Box"=0}, {"Mean"=0.0, " Std"=0.0, "Color Box"=0}, {"Mean"=0.0, " Std"=0.0, "Color Box"=0}, {"Mean"=0.0, " Std"=0.0, "Color Box"=0}, {"Mean"=0.0, " Std"=0.0, "Color Box"=0}, {"Mean"=0.0, " Std"=0.0, "Color Box"=0}, {"Mean"=0.0, " Std"=0.0, "Color Box"=0}, {"Mean"=0.0, " Std"=0.0, "Color Box"=0}, {"Mean"=0.0, " Std"=0.0, "Color Box"=0}, {"Mean"=0.0, " Std"=0.0, "Color Box"=0}, {"Mean"=0.0, " Std"=0.0, "Color Box"=0}, {"Mean"=0.0, " Std"=0.0, "Color Box"=0}, {"Mean"=0.0, " Std"=0.0, "Color Box"=0}, {"Mean"=0.0, " Std"=0.0, "Color Box"=0}, {"Mean"=0.0, " Std"=0.0, "Color Box"=0}, {"Mean"=0.0, " Std"=0.0, "Color Box"=0}, {"Mean"=0.0, " Std"=0.0, "Color Box"=0}, {"Mean"=0.0, " Std"=0.0, "Color Box"=0}, {"Mean"=0.0, " Std"=0.0, "Color Box"=0}, {"Mean"=0.0, " Std"=0.0, "Color Box"=0}, {"Mean"=0.0, " Std"=0.0, "Color Box"=0}, {"Mean"=0.0, " Std"=0.0, "Color Box"=0}, {"Mean"=0.0, " Std"=0.0, "Color Box"=0}, {"Mean"=0.0, " Std"=0.0, "Color Box"=0}, {"Mean"=0.0, " Std"=0.0, "Color Box"=0}, {"Mean"=0.0, " Std"=0.0, "Color Box"=0}, {"Mean"=0.0, " Std"=0.0, "Color Box"=0}, {"Mean"=0.0, " Std"=0.0, "Color Box"=0}, {"Mean"=0.0, " Std"=0.0, "Color Box"=0}, {"Mean"=0.0, " Std"=0.0, "Color Box"=0}, {"Mean"=0.0, " Std"=0.0, "Color Box"=0}, {"Mean"=0.0, " Std"=0.0, "Color Box"=0}, {"Mean"=0.0, " Std"=0.0, "Color Box"=0}, {"Mean"=0.0, " Std"=0.0, "Color Box"=0}, {"Mean"=0.0, " Std"=0.0, "Color Box"=0}, {"Mean"=0.0, " Std"=0.0, "Color Box"=0}, {"Mean"=0.0, " Std"=0.0, "Color Box"=0}, {"Mean"=0.0, " Std"=0.0, "Color Box"=0}, {"Mean"=0.0, " Std"=0.0, "Color Box"=0}, {"Mean"=0.0, " Std"=0.0, "Color Box"=0}, {"Mean"=0.0, " Std"=0.0, "Color Box"=0}, {"Mean"=0.0, " Std"=0.0, "Color Box"=0}, {"Mean"=0.0, " Std"=0.0, "Color Box"=0}, {"Mean"=0.0, " Std"=0.0, "Color Box"=0}, {"Mean"=0.0, " Std"=0.0, "Color Box"=0}, {"Mean"=0.0, " Std"=0.0, "Color Box"=0}, {"Mean"=0.0, " Std"=0.0, "Color Box"=0}, {"Mean"=0.0, " Std"=0.0, "Color Box"=0}, {"Mean"=0.0, " Std"=0.0, "Color Box"=0}, {"Mean"=0.0, " Std"=0.0, "Color Box"=0}, {"Mean"=0.0, " Std"=0.0, "Color Box"=0}, {"Mean"=0.0, " Std"=0.0, "Color Box"=0}, {"Mean"=0.0, " Std"=0.0, "Color Box"=0}, {"Mean"=0.0, " Std"=0.0, "Color Box"=0}, {"Mean"=0.0, " Std"=0.0, "Color Box"=0}, {"Mean"=0.0, " Std"=0.0, "Color Box"=0}, {"Mean"=0.0, " Std"=0.0, "Color Box"=0}, {"Mean"=0.0, " Std"=0.0, "Color Box"=0}, {"Mean"=0.0, " Std"=0.0, "Color Box"=0}, {"Mean"=0.0, " Std"=0.0, "Color Box"=0}, {"Mean"=0.0, " Std"=0.0, "Color Box"=0}, {"Mean"=0.0, " Std"=0.0, "Color Box"=0}, {"Mean"=0.0, " Std"=0.0, "Color Box"=0}, {"Mean"=0.0, " Std"=0.0, "Color Box"=0}, {"Mean"=0.0, " Std"=0.0, "Color Box"=0}, {"Mean"=0.0, " Std"=0.0, "Color Box"=0}, {"Mean"=0.0, " Std"=0.0, "Color Box"=0}, {"Mean"=0.0, " Std"=0.0, "Color Box"=0}, {"Mean"=0.0, " Std"=0.0, "Color Box"=0}, {"Mean"=0.0, " Std"=0.0, "Color Box"=0}, {"Mean"=0.0, " Std"=0.0, "Color Box"=0}, {"Mean"=0.0, " Std"=0.0, "Color Box"=0}, {"Mean"=0.0, " Std"=0.0, "Color Box"=0}, {"Mean"=0.0, " Std"=0.0, "Color Box"=0}, {"Mean"=0.0, " Std"=0.0, "Color Box"=0}, {"Mean"=0.0, " Std"=0.0, "Color Box"=0}, {"Mean"=0.0, " Std"=0.0, "Color Box"=0}, {"Mean"=0.0, " Std"=0.0, "Color Box"=0}, {"Mean"=0.0, " Std"=0.0, "Color Box"=0}, {"Mean"=0.0, " Std"=0.0, "Color Box"=0}, {"Mean"=0.0, " Std"=0.0, "Color Box"=0}, {"Mean"=0.0, " Std"=0.0, "Color Box"=0}, {"Mean"=0.0, " Std"=0.0, "Color Box"=0}, {"Mean"=0.0, " Std"=0.0, "Color Box"=0}, {"Mean"=0.0, " Std"=0.0, "Color Box"=0}, {"Mean"=0.0, " Std"=0.0, "Color Box"=0}, {"Mean"=0.0, " Std"=0.0, "Color Box"=0}, {"Mean"=0.0, " Std"=0.0, "Color Box"=0}, {"Mean"=0.0, " Std"=0.0, "Color Box"=0}, {"Mean"=0.0, " Std"=0.0, "Color Box"=0}, {"Mean"=0.0, " Std"=0.0, "Color Box"=0}, {"Mean"=0.0, " Std"=0.0, "Color Box"=0}, {"Mean"=0.0, " Std"=0.0, "Color Box"=0}, {"Mean"=0.0, " Std"=0.0, "Color Box"=0}, {"Mean"=0.0, " Std"=0.0, "Color Box"=0}, {"Mean"=0.0, " Std"=0.0, "Color Box"=0}, {"Mean"=0.0, " Std"=0.0, "Color Box"=0}, {"Mean"=0.0, " Std"=0.0, "Color Box"=0}, {"Mean"=0.0, " Std"=0.0, "Color Box"=0}, {"Mean"=0.0, " Std"=0.0, "Color Box"=0}, {"Mean"=0.0, " Std"=0.0, "Color Box"=0}, {"Mean"=0.0, " Std"=0.0, "Color Box"=0}, {"Mean"=0.0, " Std"=0.0, "Color Box"=0}, {"Mean"=0.0, " Std"=0.0, "Color Box"=0}, {"Mean"=0.0, " Std"=0.0, "Color Box"=0}, {"Mean"=0.0, " Std"=0.0, "Color Box"=0}, {"Mean"=0.0, " Std"=0.0, "Color Box"=0}, {"Mean"=0.0, " Std"=0.0, "Color Box"=0}, {"Mean"=0.0, " Std"=0.0, "Color Box"=0}, {"Mean"=0.0, " Std"=0.0, "Color Box"=0}, {"Mean"=0.0, " Std"=0.0, "Color Box"=0}, {"Mean"=0.0, " Std"=0.0, "Color Box"=0}, {"Mean"=0.0, " Std"=0.0, "Color Box"=0}, {"Mean"=0.0, " Std"=0.0, "Color Box"=0}, {"Mean"=0.0, " Std"=0.0, "Color Box"=0}, {"Mean"=0.0, " Std"=0.0, "Color Box"=0}, {"Mean"=0.0, " Std"=0.0, "Color Box"=0}, {"Mean"=0.0, " Std"=0.0, "Color Box"=0}, {"Mean"=0.0, " Std"=0.0, "Color Box"=0}, {"Mean"=0.0, " Std"=0.0, "Color Box"=0}, {"Mean"=0.0, " Std"=0.0, "Color Box"=0}, {"Mean"=0.0, " Std"=0.0, "Color Box"=0}, {"Mean"=0.0, " Std"=0.0, "Color Box"=0}, {"Mean"=0.0, " Std"=0.0, "Color Box"=0}, {"Mean"=0.0, " Std"=0.0, "Color Box"=0}, {"Mean"=0.0, " Std"=0.0, "Color Box"=0}, {"Mean"=0.0, " Std"=0.0, "Color Box"=0}, {"Mean"=0.0, " Std"=0.0, "Color Box"=0}, {"Mean"=0.0, " Std"=0.0, "Color Box"=0}, {"Mean"=0.0, " Std"=0.0, "Color Box"=0}, {"Mean"=0.0, " Std"=0.0, "Color Box"=0}, {"Mean"=0.0, " Std"=0.0, "Color Box"=0}, {"Mean"=0.0, " Std"=0.0, "Color Box"=0}, {"Mean"=0.0, " Std"=0.0, "Color Box"=0}, {"Mean"=0.0, " Std"=0.0, "Color Box"=0}, {"Mean"=0.0, " Std"=0.0, "Color Box"=0}, {"Mean"=0.0, " Std"=0.0, "Color Box"=0}, {"Mean"=0.0, " Std"=0.0, "Color Box"=0}, {"Mean"=0.0, " Std"=0.0, "Color Box"=0}, {"Mean"=0.0, " Std"=0.0, "Color Box"=0}, {"Mean"=0.0, " Std"=0.0, "Color Box"=0}, {"Mean"=0.0, " Std"=0.0, "Color Box"=0}, {"Mean"=0.0, " Std"=0.0, "Color Box"=0}, {"Mean"=0.0, " Std"=0.0, "Color Box"=0}, {"Mean"=0.0, " Std"=0.0, "Color Box"=0}, {"Mean"=0.0, " Std"=0.0, "Color Box"=0}, {"Mean"=0.0, " Std"=0.0, "Color Box"=0}, {"Mean"=0.0, " Std"=0.0, "Color Box"=0}, {"Mean"=0.0, " Std"=0.0, "Color Box"=0}, {"Mean"=0.0, " Std"=0.0, "Color Box"=0}, {"Mean"=0.0, " Std"=0.0, "Color Box"=0}, {"Mean"=0.0, " Std"=0.0, "Color Box"=0}, {"Mean"=0.0, " Std"=0.0, "Color Box"=0}, {"Mean"=0.0, " Std"=0.0, "Color Box"=0}, {"Mean"=0.0, " Std"=0.0, "Color Box"=0}, {"Mean"=0.0, " Std"=0.0, "Color Box"=0}, {"Mean"=0.0, " Std"=0.0, "Color Box"=0}, {"Mean"=0.0, " Std"=0.0, "Color Box"=0}, {"Mean"=0.0, " Std"=0.0, "Color Box"=0}, {"Mean"=0.0, " Std"=0.0, "Color Box"=0}, {"Mean"=0.0, " Std"=0.0, "Color Box"=0}, {"Mean"=0.0, " Std"=0.0, "Color Box"=0}, {"Mean"=0.0, " Std"=0.0, "Color Box"=0}, {"Mean"=0.0, " Std"=0.0, "Color Box"=0}, {"Mean"=0.0, " Std"=0.0, "Color Box"=0}, {"Mean"=0.0, " Std"=0.0, "Color Box"=0}, {"Mean"=0.0, " Std"=0.0, "Color Box"=0}, {"Mean"=0.0, " Std"=0.0, "Color Box"=0}, {"Mean"=0.0, " Std"=0.0, "Color Box"=0}, {"Mean"=0.0, " Std"=0.0, "Color Box"=0}, {"Mean"=0.0, " Std"=0.0, "Color Box"=0}, {"Mean"=0.0, " Std"=0.0, "Color Box"=0}, {"Mean"=0.0, " Std"=0.0, "Color Box"=0}, {"Mean"=0.0, " Std"=0.0, "Color Box"=0}, {"Mean"=0.0, " Std"=0.0, "Color Box"=0}, {"Mean"=0.0, " Std"=0.0, "Color Box"=0}, {"Mean"=0.0, " Std"=0.0, "Color Box"=0}, {"Mean"=0.0, " Std"=0.0, "Color Box"=0}, {"Mean"=0.0, " Std"=0.0, "Color Box"=0}, {"Mean"=0.0, " Std"=0.0, "Color Box"=0}, {"Mean"=0.0, " Std"=0.0, "Color Box"=0}, {"Mean"=0.0, " Std"=0.0, "Color Box"=0}, {"Mean"=0.0, " Std"=0.0, "Color Box"=0}, {"Mean"=0.0, " Std"=0.0, "Color Box"=0}, {"Mean"=0.0, " Std"=0.0, "Color Box"=0}, {"Mean"=0.0, " Std"=0.0, "Color Box"=0}, {"Mean"=0.0, " Std"=0.0, "Color Box"=0}, {"Mean"=0.0, " Std"=0.0, "Color Box"=0}, {"Mean"=0.0, " Std"=0.0, "Color Box"=0}, {"Mean"=0.0, " Std"=0.0, "Color Box"=0}, {"Mean"=0.0, " Std"=0.0, "Color Box"=0}, {"Mean"=0.0, " Std"=0.0, "Color Box"=0}, {"Mean"=0.0, " Std"=0.0, "Color Box"=0}, {"Mean"=0.0, " Std"=0.0, "Color Box"=0}, {"Mean"=0.0, " Std"=0.0, "Color Box"=0}, {"Mean"=0.0, " Std"=0.0, "Color Box"=0}, {"Mean"=0.0, " Std"=0.0, "Color Box"=0}, {"Mean"=0.0, " Std"=0.0, "Color Box"=0}, {"Mean"=0.0, " Std"=0.0, "Color Box"=0}, {"Mean"=0.0, " Std"=0.0, "Color Box"=0}, {"Mean"=0.0, " Std"=0.0, "Color Box"=0}, {"Mean"=0.0, " Std"=0.0, "Color Box"=0}, {"Mean"=0.0, " Std"=0.0, "Color Box"=0}, {"Mean"=0.0, " Std"=0.0, "Color Box"=0}, {"Mean"=0.0, " Std"=0.0, "Color Box"=0}, {"Mean"=0.0, " Std"=0.0, "Color Box"=0}, {"Mean"=0.0, " Std"=0.0, "Color Box"=0}, {"Mean"=0.0, " Std"=0.0, "Color Box"=0}, {"Mean"=0.0, " Std"=0.0, "Color Box"=0}, {"Mean"=0.0, " Std"=0.0, "Color Box"=0}, {"Mean"=0.0, " Std"=0.0, "Color Box"=0}, {"Mean"=0.0, " Std"=0.0, "Color Box"=0}, {"Mean"=0.0, " Std"=0.0, "Color Box"=0}, {"Mean"=0.0, " Std"=0.0, "Color Box"=0}, {"Mean"=0.0, " Std"=0.0, "Color Box"=0}, {"Mean"=0.0, " Std"=0.0, "Color Box"=0}, {"Mean"=0.0, " Std"=0.0, "Color Box"=0}, {"Mean"=0.0, " Std"=0.0, "Color Box"=0}, {"Mean"=0.0, " Std"=0.0, "Color Box"=0}, {"Mean"=0.0, " Std"=0.0, "Color Box"=0}, {"Mean"=0.0, " Std"=0.0, "Color Box"=0}, {"Mean"=0.0, " Std"=0.0, "Color Box"=0}, {"Mean"=0.0, " Std"=0.0, "Color Box"=0}, {"Mean"=0.0, " Std"=0.0, "Color Box"=0}, {"Mean"=0.0, " Std"=0.0, "Color Box"=0}, {"Mean"=0.0, " Std"=0.0, "Color Box"=0}, {"Mean"=0.0, " Std"=0.0, "Color Box"=0}, {"Mean"=0.0, " Std"=0.0, "Color Box"=0}, {"Mean"=0.0, " Std"=0.0, "Color Box"=0}, {"Mean"=0.0, " Std"=0.0, "Color Box"=0}, {"Mean"=0.0, " Std"=0.0, "Color Box"=0}, {"Mean"=0.0, " Std"=0.0, "Color Box"=0}, {"Mean"=0.0, " Std"=0.0, "Color Box"=0}, {"Mean"=0.0, " Std"=0.0, "Color Box"=0}, {"Mean"=0.0, " Std"=0.0, "Color Box"=0}, {"Mean"=0.0, " Std"=0.0, "Color Box"=0}, {"Mean"=0.0, " Std"=0.0, "Color Box"=0}, {"Mean"=0.0, " Std"=0.0, "Color Box"=0}, {"Mean"=0.0, " Std"=0.0, "Color Box"=0}, {"Mean"=0.0, " Std"=0.0, "Color Box"=0}, {"Mean"=0.0, " Std"=0.0, "Color Box"=0}, {"Mean"=0.0, " Std"=0.0, "Color Box"=0}, {"Mean"=0.0, " Std"=0.0, "Color Box"=0}, {"Mean"=0.0, " Std"=0.0, "Color Box"=0}, {"Mean"=0.0, " Std"=0.0, "Color Box"=0}, {"Mean"=0.0, " Std"=0.0, "Color Box"=0}, {"Mean"=0.0, " Std"=0.0, "Color Box"=0}, {"Mean"=0.0, " Std"=0.0, "Color Box"=0}, {"Mean"=0.0, " Std"=0.0, "Color Box"=0}, {"Mean"=0.0, " Std"=0.0, "Color Box"=0}, {"Mean"=0.0, " Std"=0.0, "Color Box"=0}, {"Mean"=0.0, " Std"=0.0, "Color Box"=0}, {"Mean"=0.0, " Std"=0.0, "Color Box"=0}, {"Mean"=0.0, " Std"=0.0, "Color Box"=0}, {"Mean"=0.0, " Std"=0.0, "Color Box"=0}, {"Mean"=0.0, " Std"=0.0, "Color Box"=0}, {"Mean"=0.0, " Std"=0.0, "Color Box"=0}, {"Mean"=0.0, " Std"=0.0, "Color Box"=0}, {"Mean"=0.0, " Std"=0.0, "Color Box"=0}, {"Mean"=0.0, " Std"=0.0, "Color Box"=0}, {"Mean"=0.0, " Std"=0.0, "Color Box"=0}, {"Mean"=0.0, " Std"=0.0, "Color Box"=0}, {"Mean"=0.0, " Std"=0.0, "Color Box"=0}, {"Mean"=0.0, " Std"=0.0, "Color Box"=0}, {"Mean"=0.0, " Std"=0.0, "Color Box"=0}, {"Mean"=0.0, " Std"=0.0, "Color Box"=0}, {"Mean"=0.0, " Std"=0.0, "Color Box"=0}, {"Mean"=0.0, " Std"=0.0, "Color Box"=0}, {"Mean"=0.0, " Std"=0.0, "Color Box"=0}, {"Mean"=0.0, " Std"=0.0, "Color Box"=0}, {"Mean"=0.0, " Std"=0.0, "Color Box"=0}, {"Mean"=0.0, " Std"=0.0, "Color Box"=0}, {"Mean"=0.0, " Std"=0.0, "Color Box"=0}, {"Mean"=0.0, " Std"=0.0, "Color Box"=0}, {"Mean"=0.0, " Std"=0.0, "Color Box"=0}, {"Mean"=0.0, " Std"=0.0, "Color Box"=0}, {"Mean"=0.0, " Std"=0.0, "Color Box"=0}, {"Mean"=0.0, " Std"=0.0, "Color Box"=0}, {"Mean"=0.0, " Std"=0.0, "Color Box"=0}, {"Mean"=0.0, " Std"=0.0, "Color Box"=0}, {"Mean"=0.0, " Std"=0.0, "Color Box"=0}, {"Mean"=0.0, " Std"=0.0, "Color Box"=0}, {"Mean"=0.0, " Std"=0.0, "Color Box"=0}, {"Mean"=0.0, " Std"=0.0, "Color Box"=0}, {"Mean"=0.0, " Std"=0.0, "Color Box"=0}, {"Mean"=0.0, " Std"=0.0, "Color Box"=0}, {"Mean"=0.0, " Std"=0.0, "Color Box"=0}, {"Mean"=0.0, " Std"=0.0, "Color Box"=0}, {"Mean"=0.0, " Std"=0.0, "Color Box"=0}, {"Mean"=0.0, " Std"=0.0, "Color Box"=0}, {"Mean"=0.0, " Std"=0.0, "Color Box"=0}, {"Mean"=0.0, " Std"=0.0, "Color Box"=0}, {"Mean"=0.0, " Std"=0.0, "Color Box"=0}, {"Mean"=0.0, " Std"=0.0, "Color Box"=0}, {"Mean"=0.0, " Std"=0.0, "Color Box"=0}, {"Mean"=0.0, " Std"=0.0, "Color Box"=0}, {"Mean"=0.0, " Std"=0.0, "Color Box"=0}, {"Mean"=0.0, " Std"=0.0, "Color Box"=0}, {"Mean"=0.0, " Std"=0.0, "Color Box"=0}, {"Mean"=0.0, " Std"=0.0, "Color Box"=0}, {"Mean"=0.0, " Std"=0.0, "Color Box"=0}, {"Mean"=0.0, " Std"=0.0, "Color Box"=0}, {"Mean"=0.0, " Std"=0.0, "Color Box"=0}, {"Mean"=0.0, " Std"=0.0, "Color Box"=0}, {"Mean"=0.0, " Std"=0.0, "Color Box"=0}, {"Mean"=0.0, " Std"=0.0, "Color Box"=0}, {"Mean"=0.0, " Std"=0.0, "Color Box"=0}, {"Mean"=0.0, " Std"=0.0, "Color Box"=0}, {"Mean"=0.0, " Std"=0.0, "Color Box"=0}, {"Mean"=0.0, " Std"=0.0, "Color Box"=0}, {"Mean"=0.0, " Std"=0.0, "Color Box"=0}, {"Mean"=0.0, " Std"=0.0, "Color Box"=0}, {"Mean"=0.0, " Std"=0.0, "Color Box"=0}, {"Mean"=0.0, " Std"=0.0, "Color Box"=0}, {"Mean"=0.0, " Std"=0.0, "Color Box"=0}, {"Mean"=0.0, " Std"=0.0, "Color Box"=0}, {"Mean"=0.0, " Std"=0.0, "Color Box"=0}, {"Mean"=0.0, " Std"=0.0, "Color Box"=0}, {"Mean"=0.0, " Std"=0.0, "Color Box"=0}, {"Mean"=0.0, " Std"=0.0, "Color Box"=0}, {"Mean"=0.0, " Std"=0.0, "Color Box"=0}, {"Mean"=0.0, " Std"=0.0, "Color Box"=0}, {"Mean"=0.0, " Std"=0.0, "Color Box"=0}, {"Mean"=0.0, " Std"=0.0, "Color Box"=0}, {"Mean"=0.0, " Std"=0.0, "Color Box"=0}, {"Mean"=0.0, " Std"=0.0, "Color Box"=0}, {"Mean"=0.0, " Std"=0.0, "Color Box"=0}, {"Mean"=0.0, " Std"=0.0, "Color Box"=0}, {"Mean"=0.0, " Std"=0.0, "Color Box"=0}, {"Mean"=0.0, " Std"=0.0, "Color Box"=0}, {"Mean"=0.0, " Std"=0.0, "Color Box"=0}, {"Mean"=0.0, " Std"=0.0, "Color Box"=0}, {"Mean"=0.0, " Std"=0.0, "Color Box"=0}, {"Mean"=0.0, " Std"=0.0, "Color Box"=0}, {"Mean"=0.0, " Std"=0.0, "Color Box"=0}, {"Mean"=0.0, " Std"=0.0, "Color Box"=0}, {"Mean"=0.0, " Std"=0.0, "Color Box"=0}, {"Mean"=0.0, " Std"=0.0, "Color Box"=0}, {"Mean"=0.0, " Std"=0.0, "Color Box"=0}, {"Mean"=0.0, " Std"=0.0, "Color Box"=0}, {"Mean"=0.0, " Std"=0.0, "Color Box"=0}, {"Mean"=0.0, " Std"=0.0, "Color Box"=0}, {"Mean"=0.0, " Std"=0.0, "Color Box"=0}, {"Mean"=0.0, " Std"=0.0, "Color Box"=0}, {"Mean"=0.0, " Std"=0.0, "Color Box"=0}, {"Mean"=0.0, " Std"=0.0, "Color Box"=0}, {"Mean"=0.0, " Std"=0.0, "Color Box"=0}, {"Mean"=0.0, " Std"=0.0, "Color Box"=0}]  # Temp  Data Array
        w115 = T6 {"Current VI Reference"=refnum, "Close Panel on Exit?"=FALSE}  # Core
        n38 = flat-sequence {
          tunnel: ["CDAQ Data"] -> w102
          frame #0 {
            w120 = 95  # CDAQ Array Size
            n39 = Initialize Array(0.0 ("Mean"), w120) -> (w119:dbl[])
            n40 = local write "CDAQ Data"(w119) -> ()
          }
          frame #1 {
          }
        }
        n41 = call "Cont Acq Thermocouple Samples-Int Clk-Init.vi"("error in"=w110, "Rate"=75.0) -> ("error out"=w108:errorcluster, "Temp task out"=w112:refnum<k21>)  [unwired: 8 in]
        n42 = call "Cont Acq AI Samples-Int Clk-Init.vi"("error in"=w108, "Rate"="Rate") -> ("error out"=w105:errorcluster, "AI task out"=w109:refnum<k21>)  [unwired: 8 in]
        n43 = case shown="Error" w105 {
          tunnel: [_ " Macro: Exit" ("State(s) in Front (\"\")")] -> w104
          frame #0 {
          }
          frame #1 {
          }
        }
        n44 = Bundle("Core"=w115, "Num Samples"="Num Samples", "Temp task out"=w112, "Temp  Data Array"=w113, "AI task out"=w109, "AI Data"=w107, "Init"=w103, "CDAQ Data"=w102) -> (w116:T5)  [unwired: 1 in]
        n45 = call <vilib>:"Add State(s) to Queue__jki_lib_state_machine.vi"("State(s) in Front (\"\")"=w104, "State(s) in (\"\")"=w118) -> ("States Out"=w117:string)  [unwired: 13 in]
      }
      frame #8 {
        # "Cleanup any data and references, here.\n(this is called automatically, by the Macro: Exit)"
        n46 = Unbundle By Name(w127) -> ("Core.Current VI Reference"=w129:refnum<vi>, "Temp task out"=w126:refnum<k21>)
        n47 = call <vilib>:"DAQmx Clear Task.vi"("task in"=w126, "error in"=w125) -> ("error out"=w124:errorcluster)  [unwired: 13 in]
        n48 = Close Reference(reference=w129, error in (no error)=w124) -> (error out=w128:errorcluster)
        n49 = call <vilib>:"Add State(s) to Queue__jki_lib_state_machine.vi"("State(s) in (\"\")"=w131) -> ("States Out"=w130:string)  [unwired: 14 in]
      }
      frame #9 {
        # "Do not put any code in this frame.\n(It is a separator no-op. You can make a copy of this frame to create a new UI frame)"
        n50 = call <vilib>:"Add State(s) to Queue__jki_lib_state_machine.vi"("State(s) in (\"\")"=w135) -> ("States Out"=w134:string)  [unwired: 14 in]
      }
      frame #10 {
        w140 = T2 {"Mean"=99.0, " Std"=99.0, "Color Box"=16318226} ("Sensor")
        # "Initialize the User Interface, here.\n(this is called automatically, by the Macro: Init)"
        n51 = stacked-sequence {
          tunnel: "Panel 1" -> [w148 w161]
          tunnel: w140 -> [w147 w160]
          tunnel: [w146 _] -> w137
          tunnel: "Panel 2" -> [_ _]
          tunnel: "Panel 3" -> [_ _]
          tunnel: [_ w158] -> _
          tunnel: "Panel 4" -> [_ _]
          frame #0 {
            n52 = for {
              tunnel: w148 -> [w151] mode=indexing
              tunnel: w147 -> [w150]
              tunnel: [w149] -> w146 mode=indexing
              n53 = for {
                tunnel: w151 -> [w157] mode=indexing
                tunnel: w150 -> [w156]
                tunnel: [w152] -> w149 mode=indexing
                n54 = Unbundle(w156) -> ("Mean"=w155:dbl, "Std"=w154:dbl, "Color Box"=w153:u32)
                n55 = Bundle By Name(cluster=w157, "Mean"=w155, "Color Box"=w154, "Color Box"=w153) -> (w152:T2)
              }
            }
          }
          frame #1 {
            n56 = for {
              N: 3 -> [_]
              tunnel: w161 -> [_] mode=indexing
              tunnel: w160 -> [w162]
              tunnel: [w162] -> w158 mode=indexing
            }
          }
        }
        n57 = local write "Panel 4"(w137) -> ()
        n58 = local write "Panel 1"(w137) -> ()
        n59 = local write "Panel 2"(w137) -> ()
        n60 = local write "Panel 3"(w137) -> ()
        n61 = call <vilib>:"Add State(s) to Queue__jki_lib_state_machine.vi"("State(s) in (\"\")"=w145) -> ("States Out"=w144:string)  [unwired: 14 in]
        "Gas Temp" <- w140
      }
      frame #11 {
        # "Argument"
        # "Set and Unset Cursor Busy.\n(Usage: \"UI: Cursor Set >> Busy|Idle\")"
        n62 = case shown="\"Idle\", Default" w163 {
          tunnel: w165 -> [w170 w172]
          tunnel: [w169 w171] -> w164
          frame #0 {
            n63 = call <vilib>:"Unset Busy.vi"("error in (no error)"=w170) -> ("error out"=w169:errorcluster)  [unwired: 10 in]
          }
          frame #1 {
            n64 = call <vilib>:"Set Busy.vi"("error in (no error)"=w172) -> ("error out"=w171:errorcluster)  [unwired: 9 in, 1 out]
          }
        }
        n65 = call <vilib>:"Add State(s) to Queue__jki_lib_state_machine.vi"("State(s) in (\"\")"=w168) -> ("States Out"=w167:string)  [unwired: 14 in]
      }
      frame #12 {
        # "Argument"
        # "Set Front Panel Open or Closed\n(Usage: \"UI: Front Panel State >> Open|Close\")"
        n66 = Unbundle By Name(w175) -> ("Core.Current VI Reference"=w174:refnum<vi>)
        n67 = case shown="\"Close\"" w173 {
          tunnel: w177 -> [w183 w196]
          tunnel: [w185 w197] -> w176
          tunnel: w174 -> [w184 w194]
          frame #0 {
            n68 = property class="VI"(reference=w184, error in=w183) -> (reference out=w181:refnum<vi>, error out=w182:errorcluster, "Front Panel.Open"=w180:bool)
            n69 = case shown="False" w180 {
              tunnel: [w188 w191] -> w185
              tunnel: w182 -> [w187 w191]
              tunnel: w181 -> [w186 _]
              frame #0 {
                n70 = invoke class="VI" method="FP.Open"(reference=w186, error in=w187, "Activate"=TRUE, "State"=T4."Standard") -> (error out=w188:errorcluster)  [unwired: 1 in, 4 out]
              }
              frame #1 {
              }
            }
          }
          frame #1 {
            n71 = property class="VI"(reference=w194, error in=w196) -> (reference out=w193:refnum<vi>, error out=w195:errorcluster, "Front Panel.Open"=w192:bool)
            n72 = case shown="True" w192 {
              tunnel: [w198 w201] -> w197
              tunnel: w195 -> [w198 w200]
              tunnel: w193 -> [_ w199]
              frame #0 {
              }
              frame #1 {
                n73 = invoke class="VI" method="FP.Close"(reference=w199, error in=w200) -> (error out=w201:errorcluster)  [unwired: 1 in, 2 out]
              }
            }
          }
        }
        n74 = call <vilib>:"Add State(s) to Queue__jki_lib_state_machine.vi"("State(s) in (\"\")"=w179) -> ("States Out"=w178:string)  [unwired: 14 in]
      }
      frame #13 {
        # "Do not put any code in this frame.\n(It is a separator no-op. You can make a copy of this frame to create a new Macro frame)"
        n75 = call <vilib>:"Add State(s) to Queue__jki_lib_state_machine.vi"("State(s) in (\"\")"=w205) -> ("States Out"=w204:string)  [unwired: 14 in]
      }
      frame #14 {
        # "Initialization Macro\n(This is called once, when the VI starts)"
        n76 = call <vilib>:"Add State(s) to Queue__jki_lib_state_machine.vi"("State(s) in Front (\"\")"="Data: Initialize\nInitialize Core Data\nUI: Initialize\nUI: Front Panel State >> Open", "State(s) in (\"\")"=w210) -> ("States Out"=w209:string)  [unwired: 13 in]
      }
      frame #15 {
        # "Exit Macro\n(This is called once, when the VI exits)"
        n77 = Unbundle By Name(w217) -> ("Core.Close Panel on Exit?"=w216:bool)
        n78 = Select(t="UI: Front Panel State >> Close", s=w216, f="") -> (s? t:f=w213:string)
        n79 = call <vilib>:"Add State(s) to Queue__jki_lib_state_machine.vi"("State(s) in (\"\")"=w213, "State(s) at Back (\"\")"="Data: Cleanup\nExit") -> ("States Out"=w211:string)  [unwired: 13 in]
        n80 = call <vilib>:"Add State(s) to Queue__jki_lib_state_machine.vi"("State(s) in Front (\"\")"=w211, "State(s) in (\"\")"=w220) -> ("States Out"=w219:string)  [unwired: 13 in]
      }
      frame #16 {
        # "Template Separator\n(You can make a copy of, or modify, this frame)"
        n81 = call <vilib>:"Add State(s) to Queue__jki_lib_state_machine.vi"("State(s) in (\"\")"=w224) -> ("States Out"=w223:string)  [unwired: 14 in]
      }
      frame #17 {
        # "Your code here.\n(You can make a copy of, or modify, this frame)"
        n82 = call <vilib>:"Add State(s) to Queue__jki_lib_state_machine.vi"("State(s) in (\"\")"=w229, "State(s) at Back (\"\")"="TestDAQ: Gather\nTestDAQ: Sort\nTestDAQ: Verify" ("State(s) at Back (\"\")")) -> ("States Out"=w228:string)  [unwired: 13 in]
      }
      frame #18 {
        # "Template Separator\n(You can make a copy of, or modify, this frame)"
        n83 = call <vilib>:"Add State(s) to Queue__jki_lib_state_machine.vi"("State(s) in (\"\")"=w233) -> ("States Out"=w232:string)  [unwired: 14 in]
      }
      frame #19 {
        w241 = -1 ("number of samples per channel")
        # "Template Separator\n(You can make a copy of, or modify, this frame)"
        n84 = Unbundle By Name(w250) -> ("Temp task out"=w245:refnum<k21>, "AI task out"=w242:refnum<k21>, "Init"=w236:bool)  [unwired: 1 out]
        n85 = call-poly <vilib>:"DAQmx Read.vi"("task/channels in"=w245, "number of samples per channel"=w241, "error in"=w247) -> ("data"=w246:dbl[][], "error out"=w240:errorcluster)  [unwired: 10 in, 1 out]
        n86 = call "Counter.vi"("Reset"=w236) -> ("Count"=→"Count":dbl)  [unwired: 10 in]
        n87 = call-poly <vilib>:"DAQmx Read.vi"("task/channels in"=w242, "number of samples per channel"=w241, "error in"=w240) -> ("data"=w234:dbl[][], "error out"=w239:errorcluster)  [unwired: 10 in, 1 out]
        "error gather" <- w239
        "Voltages" <- w234
        n88 = for {
          tunnel: w234 -> [w254] mode=indexing
          tunnel: [w256] -> w238 mode=indexing
          tunnel: cluster{"Mean":dbl, "StdDev":dbl} {"Mean"=0.0, "StdDev"=0.0} -> [w255]
          n89 = call <vilib>:"Std Deviation and Variance.vi"("X"=w254) -> ("mean"=w258:dbl, "standard deviation"=w257:dbl)  [unwired: 1 in, 1 out]
          n90 = Array Size(array=w254) -> (size(s)=→"Analog Samples":i32)
          n91 = Bundle By Name(cluster=w255, "Mean"=w258, "StdDev"=w257) -> (w256:cluster{"Mean":dbl, "StdDev":dbl})
        }
        n92 = call <vilib>:"Clear Errors.vi"("error in (no error)"=w239) -> ("error out"=w244:errorcluster)  [unwired: 6 in]
        n93 = for {
          tunnel: w246 -> [w263] mode=indexing
          tunnel: [w260] -> w249 mode=indexing
          n94 = call <vilib>:"Std Deviation and Variance.vi"("X"=w263) -> ("mean"=w262:dbl, "standard deviation"=w261:dbl)  [unwired: 1 in, 1 out]
          n95 = Bundle By Name(cluster=T2 {"Mean"=0.0, " Std"=0.0, "Color Box"=5373696} ("Sensor"), "Mean"=w262, "Std"=w261) -> (w260:T2)
        }
        n96 = Bundle By Name(cluster=w250, "Init"=FALSE, "Temp  Data Array"=w249, "AI Data"=w238) -> (w248:T5)
        n97 = call <vilib>:"Add State(s) to Queue__jki_lib_state_machine.vi"("State(s) in (\"\")"=w252) -> ("States Out"=w251:string)  [unwired: 14 in]
      }
      frame #20 {
        # "Gs Pressure 0\nWeight 1\nRH 2\nGas Volume 3\nTemp 4\nBaromentric Pressure 5"
        # "Template Separator\n(You can make a copy of, or modify, this frame)"
        n98 = global read "Global Test Variables DPT.vi" "Globals for Dryer Performance Test"() -> (w274:T7)
        n99 = Unbundle By Name(w274) -> ("cDAQ Array Locations.Gas Pressure"=w270:string, "cDAQ Array Locations.RH Chan"=w269:string, "cDAQ Array Locations.Temp Chan"=w268:string, "cDAQ Array Locations.Barometric Pressure"=w267:string, "cDAQ Array Locations.Gas Feedback Chan"=w266:string, "cDAQ Array Locations.Scale Channel"=w265:string)
        n100 = Unbundle By Name(w273) -> ("CDAQ Data"=w271:dbl[], "Temp  Data Array"=w276:T2[], "AI Data"=w275:cluster{"Mean":dbl, "StdDev":dbl}[])
        n101 = stacked-sequence {
          seq-local: [_ _ _ _ _ _ _ w412 _] -> [_ _ _ _ _ _ _ _ w476]
          tunnel: w276 -> [w285 w302 w319 w336 w352 _ _ _ _]
          tunnel: w275 -> [_ _ _ _ _ w388 w411 _ _]
          tunnel: w271 -> [_ _ _ _ _ _ _ w425 _]
          tunnel: w270 -> [_ _ _ _ _ _ _ _ w475]
          tunnel: w269 -> [_ _ _ _ _ _ _ _ w468]
          tunnel: w268 -> [_ _ _ _ _ _ _ _ w455]
          tunnel: w267 -> [_ _ _ _ _ _ _ _ w454]
          tunnel: w266 -> [_ _ _ _ _ _ _ _ w453]
          tunnel: w265 -> [_ _ _ _ _ _ _ _ w452]
          tunnel: [_ _ _ _ _ _ _ _ w451] -> w264
          frame #0 {
            n102 = local read "Panel 1"() -> (w282:T2[][])
            n103 = Array Subset(array=w285, index=1, length=6) -> (w284:T2[])
            n104 = Array Subset(array=w285, index=7, length=6) -> (w281:T2[])
            n105 = Array Subset(array=w285, index=13, length=3) -> (w280:T2[])
            n106 = Replace Array Subset(array=w282, new element=w284, index (row)=0) -> (w294:T2[][])  [unwired: 1 in]
            n107 = Replace Array Subset(array=w294, new element=w281, index (row)=1) -> (w292:T2[][])  [unwired: 1 in]
            n108 = Replace Array Subset(array=w292, new element=w280, index (row)=2) -> (w283:T2[][])  [unwired: 1 in]
            n109 = local write "Panel 1"(w283) -> ()
          }
          frame #1 {
            n110 = local read "Panel 2"() -> (w298:T2[][])
            n111 = Array Subset(array=w302, index=16, length=6) -> (w301:T2[])
            n112 = Array Subset(array=w302, index=22, length=6) -> (w300:T2[])
            n113 = Array Subset(array=w302, index=28, length=4) -> (w299:T2[])
            n114 = Replace Array Subset(array=w298, new element=w301, index (row)=0) -> (w311:T2[][])  [unwired: 1 in]
            n115 = Replace Array Subset(array=w311, new element=w300, index (row)=1) -> (w309:T2[][])  [unwired: 1 in]
            n116 = Replace Array Subset(array=w309, new element=w299, index (row)=2) -> (w297:T2[][])  [unwired: 1 in]
            n117 = local write "Panel 2"(w297) -> ()
          }
          frame #2 {
            n118 = local read "Panel 3"() -> (w315:T2[][])
            n119 = Array Subset(array=w319, index=32, length=6) -> (w318:T2[])
            n120 = Array Subset(array=w319, index=38, length=6) -> (w317:T2[])
            n121 = Array Subset(array=w319, index=44, length=4) -> (w316:T2[])
            n122 = Replace Array Subset(array=w315, new element=w318, index (row)=0) -> (w328:T2[][])  [unwired: 1 in]
            n123 = Replace Array Subset(array=w328, new element=w317, index (row)=1) -> (w326:T2[][])  [unwired: 1 in]
            n124 = Replace Array Subset(array=w326, new element=w316, index (row)=2) -> (w314:T2[][])  [unwired: 1 in]
            n125 = local write "Panel 3"(w314) -> ()
          }
          frame #3 {
            n126 = local read "Panel 4"() -> (w332:T2[][])
            n127 = Array Subset(array=w336, index=48, length=6) -> (w335:T2[])
            n128 = Array Subset(array=w336, index=54, length=6) -> (w334:T2[])
            n129 = Array Subset(array=w336, index=60, length=4) -> (w333:T2[])
            n130 = Replace Array Subset(array=w332, new element=w335, index (row)=0) -> (w345:T2[][])  [unwired: 1 in]
            n131 = Replace Array Subset(array=w345, new element=w334, index (row)=1) -> (w343:T2[][])  [unwired: 1 in]
            n132 = Replace Array Subset(array=w343, new element=w333, index (row)=2) -> (w331:T2[][])  [unwired: 1 in]
            n133 = local write "Panel 4"(w331) -> ()
          }
          frame #4 {
            n134 = Index Array(array=w352, index #1=35 ("index"), index #2=33 ("index"), index #3=34 ("length")) -> ()  [unwired: 3 out]
            n135 = Array Subset(array=w352, index=17, length=3) -> ()  [unwired: 1 out]
            n136 = Index Array(array=w352, index=0) -> (element=w351:T2)
            n137 = Index Array(array=w352, index=15) -> ()  [unwired: 1 out]
            n138 = local write "Gas Temp"(w351) -> ()
          }
          frame #5 {
            w369 = 250.0 ("Drop resistor")
            n139 = call "Scale 4-20 sig.vi"("4 mA value"=0.0, "20 mA value"=50.0, "Drop resistor"=w369) -> ("M"=w386:dbl, "B"=w368:dbl)  [unwired: 11 in]
            n140 = call "Scale 4-20 sig.vi"("4 mA value"=0.0, "20 mA value"=100.0, "Drop resistor"=w369) -> ("M"=w380:dbl, "B"=w364:dbl)  [unwired: 11 in]
            n141 = call "Scale 4-20 sig.vi"("4 mA value"=32.0, "20 mA value"=212.0, "Drop resistor"=w369) -> ("M"=w372:dbl, "B"=w358:dbl)  [unwired: 11 in]
            n142 = Index Array(array=w388, index #1="I.Gas Pressure", index #2="I.RH", index #3="I.Tmp") -> (element #1=w385:cluster{"Mean":dbl, "StdDev":dbl}, element #2=w379:cluster{"Mean":dbl, "StdDev":dbl}, element #3=w370:cluster{"Mean":dbl, "StdDev":dbl})
            n143 = Multiply(x=w379, y=w380) -> (x*y=w362:cluster{"Mean":dbl, "StdDev":dbl})
            n144 = Multiply(x=w370, y=w372) -> (x*y=w359:cluster{"Mean":dbl, "StdDev":dbl})
            n145 = Multiply(x=w385, y=w386) -> (x*y=w367:cluster{"Mean":dbl, "StdDev":dbl})
            n146 = Bundle(cluster=w362, "Mean"=w364, "StdDev"=0.0) -> (w363:cluster{"Mean":dbl, "StdDev":dbl})
            n147 = Bundle(cluster=w359, "Mean"=w358, "StdDev"=0.0) -> (w360:cluster{"Mean":dbl, "StdDev":dbl})
            n148 = Bundle(cluster=w367, "Mean"=w368, "StdDev"=0.0) -> (w366:cluster{"Mean":dbl, "StdDev":dbl})
            n149 = Add(x=w367, y=w366) -> (x+y=→"G.Pres.":cluster{"Mean":dbl, "StdDev":dbl})
            n150 = Add(x=w362, y=w363) -> (x+y=→"RH":cluster{"Mean":dbl, "StdDev":dbl})
            n151 = Add(x=w359, y=w360) -> (x+y=→"Temp":cluster{"Mean":dbl, "StdDev":dbl})
          }
          frame #6 {
            n152 = Index Array(array=w411, index #1="I.Bar", index #2="I.Gvol", index #3="I.W") -> (element #1=w409:cluster{"Mean":dbl, "StdDev":dbl}, element #2=w406:cluster{"Mean":dbl, "StdDev":dbl}, element #3=w403:cluster{"Mean":dbl, "StdDev":dbl})
            n153 = Multiply(x=w409, y=1.5 ("4 mA value")) -> (x*y=w399:cluster{"Mean":dbl, "StdDev":dbl})
            n154 = Multiply(x=w406, y=1.0 ("4 mA value")) -> (x*y=w407:cluster{"Mean":dbl, "StdDev":dbl})
            n155 = Multiply(x=w403, y=15.0 ("4 mA value")) -> (x*y=w389:cluster{"Mean":dbl, "StdDev":dbl})
            n156 = Add(x=w407, y=0.0 ("4 mA value")) -> (x+y=w394:cluster{"Mean":dbl, "StdDev":dbl})
            "G.Vol" <- w394
            n157 = Bundle(cluster=w399, "Mean"=20.0 ("4 mA value"), "StdDev"=0.0) -> (w396:cluster{"Mean":dbl, "StdDev":dbl})
            n158 = Bundle(cluster=w394, "Mean"=50.0 ("4 mA value"), "StdDev"=0.0) -> (w391:cluster{"Mean":dbl, "StdDev":dbl})
            n159 = Add(x=w399, y=w396) -> (x+y=→"Bar":cluster{"Mean":dbl, "StdDev":dbl})
            n160 = Add(x=w389, y=w391) -> (x+y=→"Weight":cluster{"Mean":dbl, "StdDev":dbl})
          }
          frame #7 {
            n161 = local read "Panel 1"() -> (w426:T2[][])
            n162 = local read "Panel 2"() -> (w422:T2[][])
            n163 = local read "Panel 3"() -> (w420:T2[][])
            n164 = local read "Panel 4"() -> (w418:T2[][])
            n165 = for {
              tunnel: w426 -> [w448] mode=indexing
              shift-right: [w446] -> w414
              shift-left: dbl[] [] -> [w445]
              n166 = for {
                tunnel: w448 -> [w450] mode=indexing
                tunnel: [w449] -> w447 mode=indexing
                n167 = Unbundle By Name(w450) -> ("Mean"=w449:dbl)
              }
              n168 = Build Array (concatenate)(w445, w447) -> (w446:dbl[])
            }
            n169 = for {
              tunnel: w422 -> [w442] mode=indexing
              shift-right: [w440] -> w417
              shift-left: dbl[] [] -> [w439]
              n170 = for {
                tunnel: w442 -> [w444] mode=indexing
                tunnel: [w443] -> w441 mode=indexing
                n171 = Unbundle By Name(w444) -> ("Mean"=w443:dbl)
              }
              n172 = Build Array (concatenate)(w439, w441) -> (w440:dbl[])
            }
            n173 = for {
              tunnel: w420 -> [w436] mode=indexing
              shift-right: [w434] -> w416
              shift-left: dbl[] [] -> [w433]
              n174 = for {
                tunnel: w436 -> [w438] mode=indexing
                tunnel: [w437] -> w435 mode=indexing
                n175 = Unbundle By Name(w438) -> ("Mean"=w437:dbl)
              }
              n176 = Build Array (concatenate)(w433, w435) -> (w434:dbl[])
            }
            n177 = for {
              tunnel: w418 -> [w430] mode=indexing
              shift-right: [w428] -> w415
              shift-left: _ -> [w427]
              n178 = for {
                tunnel: w430 -> [w432] mode=indexing
                tunnel: [w431] -> w429 mode=indexing
                n179 = Unbundle By Name(w432) -> ("Mean"=w431:dbl)
              }
              n180 = Build Array (concatenate)(w427, w429) -> (w428:dbl[])
            }
            n181 = Build Array (concatenate)(w414, w417, w416, w415) -> (w413:dbl[])
            n182 = Replace Array Subset(array=w425, new element=w413, index=0) -> (w412:dbl[])
          }
          frame #8 {
            n183 = local read "G.Pres."() -> (w473:cluster{"Mean":dbl, "StdDev":dbl})
            n184 = local read "Weight"() -> (w456:cluster{"Mean":dbl, "StdDev":dbl})
            n185 = local read "Temp"() -> (w459:cluster{"Mean":dbl, "StdDev":dbl})
            n186 = local read "G.Vol"() -> (w457:cluster{"Mean":dbl, "StdDev":dbl})
            n187 = local read "Bar"() -> (w458:cluster{"Mean":dbl, "StdDev":dbl})
            n188 = local read "RH"() -> (w469:cluster{"Mean":dbl, "StdDev":dbl})
            n189 = Decimal String To Number(string=w475) -> (number=w474:i32)  [unwired: 2 in, 1 out]
            n190 = Unbundle By Name(w469) -> ("Mean"=w471:dbl)
            n191 = Unbundle By Name(w473) -> ("Mean"=w472:dbl)
            n192 = Decimal String To Number(string=w468) -> (number=w470:i32)  [unwired: 2 in, 1 out]
            n193 = Unbundle By Name(w457) -> ("Mean"=w466:dbl)
            n194 = Unbundle By Name(w459) -> ("Mean"=w464:dbl)
            n195 = Unbundle By Name(w458) -> ("Mean"=w465:dbl)
            n196 = Decimal String To Number(string=w453) -> (number=w461:i32)  [unwired: 2 in, 1 out]
            n197 = Decimal String To Number(string=w455) -> (number=w463:i32)  [unwired: 2 in, 1 out]
            n198 = Decimal String To Number(string=w454) -> (number=w462:i32)  [unwired: 2 in, 1 out]
            n199 = Unbundle By Name(w456) -> ("Mean"=w467:dbl)
            n200 = Decimal String To Number(string=w452) -> (number=w460:i32)  [unwired: 2 in, 1 out]
            n201 = Replace Array Subset(array=w476, new element #1=w472, index #1=w474, new element #2=w471, index #2=w470, new element #3=w464, index #3=w463, new element #4=w465, index #4=w462, new element #5=w466, index #5=w461, new element #6=w467, index #6=w460) -> (w451:dbl[])
          }
        }
        n202 = Bundle By Name(cluster=w273, "CDAQ Data"=w264) -> (w272:T5)
        n203 = call <vilib>:"Add State(s) to Queue__jki_lib_state_machine.vi"("State(s) in (\"\")"=w279) -> ("States Out"=w278:string)  [unwired: 14 in]
      }
      frame #21 {
        # "Template Separator\n(You can make a copy of, or modify, this frame)"
        n204 = local read "Panel 4"() -> (w480:T2[][])
        n205 = local read "Panel 3"() -> (w481:T2[][])
        n206 = local read "Panel 1"() -> (w483:T2[][])
        n207 = local read "Panel 2"() -> (w482:T2[][])
        n208 = stacked-sequence {
          tunnel: w482 -> [_ w497 _ _]
          tunnel: w483 -> [w491 _ _ _]
          tunnel: w481 -> [_ _ w502 _]
          tunnel: w480 -> [_ _ _ w507]
          tunnel: "TC Min OK Val" -> [w490 w493 w498 w503]
          tunnel: "TC Max OK Val" -> [w489 w494 w499 w504]
          tunnel: "StDev Thresh" -> [w488 w495 w500 w505]
          frame #0 {
            n209 = call "Panel Color Set.vi"("TC Min OK Val"=w490, "TC Max OK Val"=w489, "StDev Thresh"=w488, "Panel 1"=w491) -> ("Panel Out"=w492:T2[][])
            n210 = local write "Panel 1"(w492) -> ()
          }
          frame #1 {
            n211 = call "Panel Color Set.vi"("TC Min OK Val"=w493, "TC Max OK Val"=w494, "StDev Thresh"=w495, "Panel 1"=w497) -> ("Panel Out"=w496:T2[][])
            n212 = local write "Panel 2"(w496) -> ()
          }
          frame #2 {
            n213 = call "Panel Color Set.vi"("TC Min OK Val"=w498, "TC Max OK Val"=w499, "StDev Thresh"=w500, "Panel 1"=w502) -> ("Panel Out"=w501:T2[][])
            n214 = local write "Panel 3"(w501) -> ()
          }
          frame #3 {
            n215 = call "Panel Color Set.vi"("TC Min OK Val"=w503, "TC Max OK Val"=w504, "StDev Thresh"=w505, "Panel 1"=w507) -> ("Panel Out"=w506:T2[][])
            n216 = local write "Panel 4"(w506) -> ()
          }
        }
        n217 = call <vilib>:"Add State(s) to Queue__jki_lib_state_machine.vi"("State(s) in (\"\")"=w487) -> ("States Out"=w486:string)  [unwired: 14 in]
      }
    }
  }
  "error out" <- w3
  n218 = while {
    stop <- "End" stop-if-true
    n219 = event shown="[0] Timeout" {
      selector: _ -> [_]
      dyn-events: _ -> [_]
      timeout: 150 -> [_]
      event [0] Timeout {
        n220 = event-data() -> ()  [unwired: 1 in, 2 out]
      }
    }
  }
  n221 = Unbundle By Name(w2) -> ("CDAQ Data"=→"CDAQ Data Out":dbl[])
